vi "Hard.vi"() -> ()   [LabVIEW 2014]
uses:
  <vilib>/Utility/inputDevices.llb/keyboardAcquire.vi
  <vilib>/Utility/inputDevices.llb/closeKeyboard.vi
panel:
  out "Vx 2":i32
  out "x觸及位置 2":i32
  out "X障礙 2":bool
  out "y觸及位置 2":i32
  out "Vy 2":i32
  out "Y障礙 2":bool
  out "Å]YÄ²":i32
  out "Å]XÄ²":i32
  out "Å]Vy":i64
  out "Å]Vx":i32
  out "魔王":bool
  out "終點":bool
  out "遊玩時間":i32
  out "X障礙":bool
  out "Y位置 2":i32
  out "x位置 2":i32
  out "X":dbl
  out "Y":dbl
  out "小精靈":bool
  out "x位置":i32
  out "Y位置":i32
  out "Y障礙":bool
  out "x觸及位置":i32
  out "y觸及位置":i32
  out "x-y":u32
  out "Vy":i32
  out "Vx":i32
  # "小精靈"
  # "500"
  # "障礙"
  # "400"
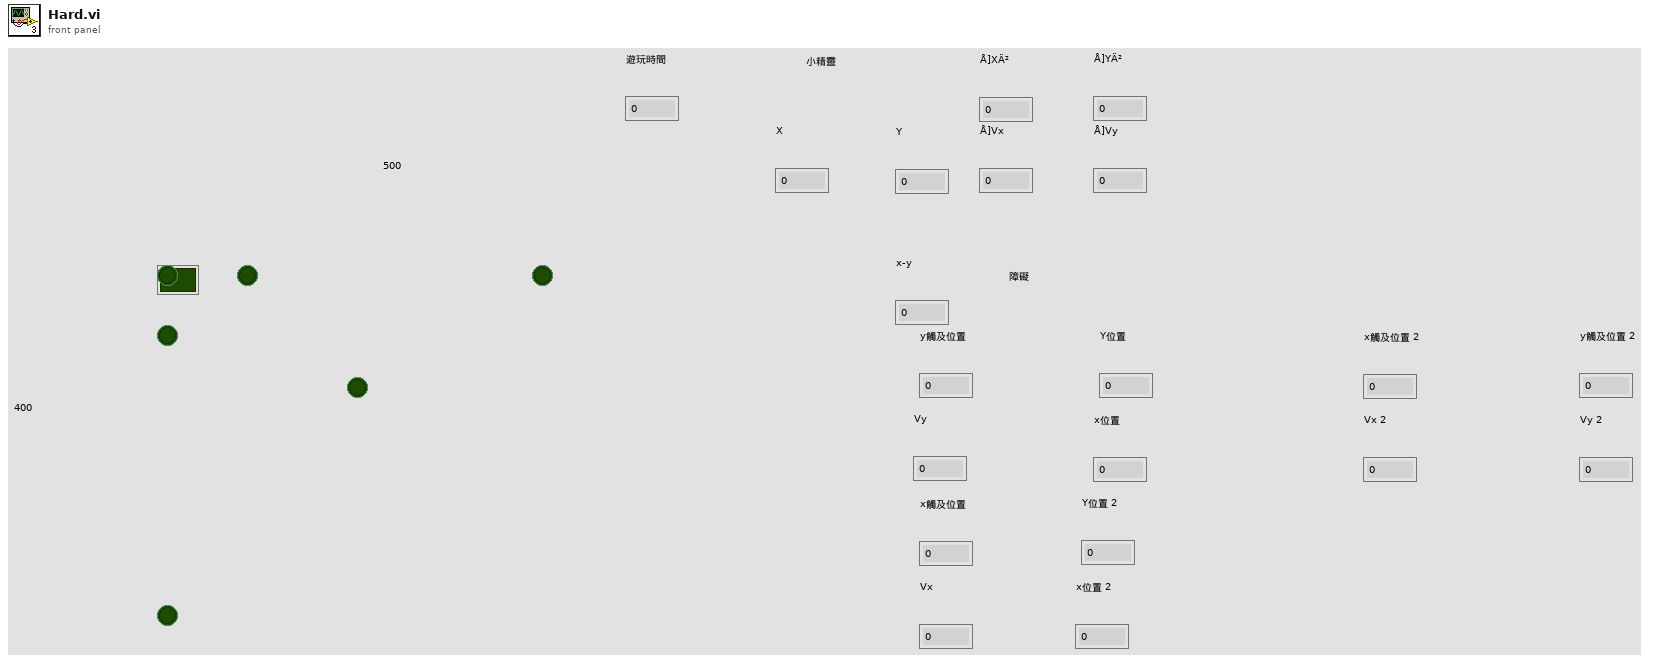
[diagram p1: front panel]
types:
  T1 = enum16{"0", "1", "2", "3", "4", "5", "6", "7", "8", "9", "A", "B", "C", "D", "E", "F", "G", "H", "I", "J", "K", "L", "M", "N", "O", "P", "Q", "R", "S", "T", "U", "V", "W", "X", "Y", "Z", "F1", "F2", "F3", "F4", "F5", "F6", "F7", "F8", "F9", "F10", "F11", "F12", "F13", "F14", "F15", "ADD", "BACK", "BACKSLASH", "CAPITAL", "COMMA", "DECIMAL", "DELETE", "DIVIDE", "DOWN", "END", "EQUALS", "ESCAPE", "GRAVE (`)", "HOME", "INSERT", "LBRACKET", "LCONTROL", "LEFT", "L ALT", "LSHIFT", "LWIN", "MINUS", "MULTIPLY", "NEXT", "NUMLOCK", "NUMPAD_0", "NUMPAD_1", "NUMPAD_2", "NUMPAD_3", "NUMPAD_4", "NUMPAD_5", "NUMPAD_6", "NUMPAD_7", "NUMPAD_8", "NUMPAD_9", "PAUSE", "PERIOD", "PRIOR (PG UP)", "RBRACKET", "RCONTROL", "RETURN", "RIGHT", "R ALT", "RSHIFT", "RWIN", "SCROLL", "SEMICOLON", "SLASH", "SPACE", "SUBTRACT", "TAB", "UP", "ENTER (num pad)", "' (quote)"}[]
  T2 = cluster{"keys pressed[0]":enum16{"0", "1", "2", "3", "4", "5", "6", "7", "8", "9", "A", "B", "C", "D", "E", "F", "G", "H", "I", "J", "K", "L", "M", "N", "O", "P", "Q", "R", "S", "T", "U", "V", "W", "X", "Y", "Z", "F1", "F2", "F3", "F4", "F5", "F6", "F7", "F8", "F9", "F10", "F11", "F12", "F13", "F14", "F15", "ADD", "BACK", "BACKSLASH", "CAPITAL", "COMMA", "DECIMAL", "DELETE", "DIVIDE", "DOWN", "END", "EQUALS", "ESCAPE", "GRAVE (`)", "HOME", "INSERT", "LBRACKET", "LCONTROL", "LEFT", "L ALT", "LSHIFT", "LWIN", "MINUS", "MULTIPLY", "NEXT", "NUMLOCK", "NUMPAD_0", "NUMPAD_1", "NUMPAD_2", "NUMPAD_3", "NUMPAD_4", "NUMPAD_5", "NUMPAD_6", "NUMPAD_7", "NUMPAD_8", "NUMPAD_9", "PAUSE", "PERIOD", "PRIOR (PG UP)", "RBRACKET", "RCONTROL", "RETURN", "RIGHT", "R ALT", "RSHIFT", "RWIN", "SCROLL", "SEMICOLON", "SLASH", "SPACE", "SUBTRACT", "TAB", "UP", "ENTER (num pad)", "' (quote)"}, "keys pressed[1]":enum16{"0", "1", "2", "3", "4", "5", "6", "7", "8", "9", "A", "B", "C", "D", "E", "F", "G", "H", "I", "J", "K", "L", "M", "N", "O", "P", "Q", "R", "S", "T", "U", "V", "W", "X", "Y", "Z", "F1", "F2", "F3", "F4", "F5", "F6", "F7", "F8", "F9", "F10", "F11", "F12", "F13", "F14", "F15", "ADD", "BACK", "BACKSLASH", "CAPITAL", "COMMA", "DECIMAL", "DELETE", "DIVIDE", "DOWN", "END", "EQUALS", "ESCAPE", "GRAVE (`)", "HOME", "INSERT", "LBRACKET", "LCONTROL", "LEFT", "L ALT", "LSHIFT", "LWIN", "MINUS", "MULTIPLY", "NEXT", "NUMLOCK", "NUMPAD_0", "NUMPAD_1", "NUMPAD_2", "NUMPAD_3", "NUMPAD_4", "NUMPAD_5", "NUMPAD_6", "NUMPAD_7", "NUMPAD_8", "NUMPAD_9", "PAUSE", "PERIOD", "PRIOR (PG UP)", "RBRACKET", "RCONTROL", "RETURN", "RIGHT", "R ALT", "RSHIFT", "RWIN", "SCROLL", "SEMICOLON", "SLASH", "SPACE", "SUBTRACT", "TAB", "UP", "ENTER (num pad)", "' (quote)"}, "keys pressed[2]":enum16{"0", "1", "2", "3", "4", "5", "6", "7", "8", "9", "A", "B", "C", "D", "E", "F", "G", "H", "I", "J", "K", "L", "M", "N", "O", "P", "Q", "R", "S", "T", "U", "V", "W", "X", "Y", "Z", "F1", "F2", "F3", "F4", "F5", "F6", "F7", "F8", "F9", "F10", "F11", "F12", "F13", "F14", "F15", "ADD", "BACK", "BACKSLASH", "CAPITAL", "COMMA", "DECIMAL", "DELETE", "DIVIDE", "DOWN", "END", "EQUALS", "ESCAPE", "GRAVE (`)", "HOME", "INSERT", "LBRACKET", "LCONTROL", "LEFT", "L ALT", "LSHIFT", "LWIN", "MINUS", "MULTIPLY", "NEXT", "NUMLOCK", "NUMPAD_0", "NUMPAD_1", "NUMPAD_2", "NUMPAD_3", "NUMPAD_4", "NUMPAD_5", "NUMPAD_6", "NUMPAD_7", "NUMPAD_8", "NUMPAD_9", "PAUSE", "PERIOD", "PRIOR (PG UP)", "RBRACKET", "RCONTROL", "RETURN", "RIGHT", "R ALT", "RSHIFT", "RWIN", "SCROLL", "SEMICOLON", "SLASH", "SPACE", "SUBTRACT", "TAB", "UP", "ENTER (num pad)", "' (quote)"}, "keys pressed[3]":enum16{"0", "1", "2", "3", "4", "5", "6", "7", "8", "9", "A", "B", "C", "D", "E", "F", "G", "H", "I", "J", "K", "L", "M", "N", "O", "P", "Q", "R", "S", "T", "U", "V", "W", "X", "Y", "Z", "F1", "F2", "F3", "F4", "F5", "F6", "F7", "F8", "F9", "F10", "F11", "F12", "F13", "F14", "F15", "ADD", "BACK", "BACKSLASH", "CAPITAL", "COMMA", "DECIMAL", "DELETE", "DIVIDE", "DOWN", "END", "EQUALS", "ESCAPE", "GRAVE (`)", "HOME", "INSERT", "LBRACKET", "LCONTROL", "LEFT", "L ALT", "LSHIFT", "LWIN", "MINUS", "MULTIPLY", "NEXT", "NUMLOCK", "NUMPAD_0", "NUMPAD_1", "NUMPAD_2", "NUMPAD_3", "NUMPAD_4", "NUMPAD_5", "NUMPAD_6", "NUMPAD_7", "NUMPAD_8", "NUMPAD_9", "PAUSE", "PERIOD", "PRIOR (PG UP)", "RBRACKET", "RCONTROL", "RETURN", "RIGHT", "R ALT", "RSHIFT", "RWIN", "SCROLL", "SEMICOLON", "SLASH", "SPACE", "SUBTRACT", "TAB", "UP", "ENTER (num pad)", "' (quote)"}, "keys pressed[4]":enum16{"0", "1", "2", "3", "4", "5", "6", "7", "8", "9", "A", "B", "C", "D", "E", "F", "G", "H", "I", "J", "K", "L", "M", "N", "O", "P", "Q", "R", "S", "T", "U", "V", "W", "X", "Y", "Z", "F1", "F2", "F3", "F4", "F5", "F6", "F7", "F8", "F9", "F10", "F11", "F12", "F13", "F14", "F15", "ADD", "BACK", "BACKSLASH", "CAPITAL", "COMMA", "DECIMAL", "DELETE", "DIVIDE", "DOWN", "END", "EQUALS", "ESCAPE", "GRAVE (`)", "HOME", "INSERT", "LBRACKET", "LCONTROL", "LEFT", "L ALT", "LSHIFT", "LWIN", "MINUS", "MULTIPLY", "NEXT", "NUMLOCK", "NUMPAD_0", "NUMPAD_1", "NUMPAD_2", "NUMPAD_3", "NUMPAD_4", "NUMPAD_5", "NUMPAD_6", "NUMPAD_7", "NUMPAD_8", "NUMPAD_9", "PAUSE", "PERIOD", "PRIOR (PG UP)", "RBRACKET", "RCONTROL", "RETURN", "RIGHT", "R ALT", "RSHIFT", "RWIN", "SCROLL", "SEMICOLON", "SLASH", "SPACE", "SUBTRACT", "TAB", "UP", "ENTER (num pad)", "' (quote)"}, "keys pressed[5]":enum16{"0", "1", "2", "3", "4", "5", "6", "7", "8", "9", "A", "B", "C", "D", "E", "F", "G", "H", "I", "J", "K", "L", "M", "N", "O", "P", "Q", "R", "S", "T", "U", "V", "W", "X", "Y", "Z", "F1", "F2", "F3", "F4", "F5", "F6", "F7", "F8", "F9", "F10", "F11", "F12", "F13", "F14", "F15", "ADD", "BACK", "BACKSLASH", "CAPITAL", "COMMA", "DECIMAL", "DELETE", "DIVIDE", "DOWN", "END", "EQUALS", "ESCAPE", "GRAVE (`)", "HOME", "INSERT", "LBRACKET", "LCONTROL", "LEFT", "L ALT", "LSHIFT", "LWIN", "MINUS", "MULTIPLY", "NEXT", "NUMLOCK", "NUMPAD_0", "NUMPAD_1", "NUMPAD_2", "NUMPAD_3", "NUMPAD_4", "NUMPAD_5", "NUMPAD_6", "NUMPAD_7", "NUMPAD_8", "NUMPAD_9", "PAUSE", "PERIOD", "PRIOR (PG UP)", "RBRACKET", "RCONTROL", "RETURN", "RIGHT", "R ALT", "RSHIFT", "RWIN", "SCROLL", "SEMICOLON", "SLASH", "SPACE", "SUBTRACT", "TAB", "UP", "ENTER (num pad)", "' (quote)"}, "keys pressed[6]":enum16{"0", "1", "2", "3", "4", "5", "6", "7", "8", "9", "A", "B", "C", "D", "E", "F", "G", "H", "I", "J", "K", "L", "M", "N", "O", "P", "Q", "R", "S", "T", "U", "V", "W", "X", "Y", "Z", "F1", "F2", "F3", "F4", "F5", "F6", "F7", "F8", "F9", "F10", "F11", "F12", "F13", "F14", "F15", "ADD", "BACK", "BACKSLASH", "CAPITAL", "COMMA", "DECIMAL", "DELETE", "DIVIDE", "DOWN", "END", "EQUALS", "ESCAPE", "GRAVE (`)", "HOME", "INSERT", "LBRACKET", "LCONTROL", "LEFT", "L ALT", "LSHIFT", "LWIN", "MINUS", "MULTIPLY", "NEXT", "NUMLOCK", "NUMPAD_0", "NUMPAD_1", "NUMPAD_2", "NUMPAD_3", "NUMPAD_4", "NUMPAD_5", "NUMPAD_6", "NUMPAD_7", "NUMPAD_8", "NUMPAD_9", "PAUSE", "PERIOD", "PRIOR (PG UP)", "RBRACKET", "RCONTROL", "RETURN", "RIGHT", "R ALT", "RSHIFT", "RWIN", "SCROLL", "SEMICOLON", "SLASH", "SPACE", "SUBTRACT", "TAB", "UP", "ENTER (num pad)", "' (quote)"}, "keys pressed[7]":enum16{"0", "1", "2", "3", "4", "5", "6", "7", "8", "9", "A", "B", "C", "D", "E", "F", "G", "H", "I", "J", "K", "L", "M", "N", "O", "P", "Q", "R", "S", "T", "U", "V", "W", "X", "Y", "Z", "F1", "F2", "F3", "F4", "F5", "F6", "F7", "F8", "F9", "F10", "F11", "F12", "F13", "F14", "F15", "ADD", "BACK", "BACKSLASH", "CAPITAL", "COMMA", "DECIMAL", "DELETE", "DIVIDE", "DOWN", "END", "EQUALS", "ESCAPE", "GRAVE (`)", "HOME", "INSERT", "LBRACKET", "LCONTROL", "LEFT", "L ALT", "LSHIFT", "LWIN", "MINUS", "MULTIPLY", "NEXT", "NUMLOCK", "NUMPAD_0", "NUMPAD_1", "NUMPAD_2", "NUMPAD_3", "NUMPAD_4", "NUMPAD_5", "NUMPAD_6", "NUMPAD_7", "NUMPAD_8", "NUMPAD_9", "PAUSE", "PERIOD", "PRIOR (PG UP)", "RBRACKET", "RCONTROL", "RETURN", "RIGHT", "R ALT", "RSHIFT", "RWIN", "SCROLL", "SEMICOLON", "SLASH", "SPACE", "SUBTRACT", "TAB", "UP", "ENTER (num pad)", "' (quote)"}, "keys pressed[8]":enum16{"0", "1", "2", "3", "4", "5", "6", "7", "8", "9", "A", "B", "C", "D", "E", "F", "G", "H", "I", "J", "K", "L", "M", "N", "O", "P", "Q", "R", "S", "T", "U", "V", "W", "X", "Y", "Z", "F1", "F2", "F3", "F4", "F5", "F6", "F7", "F8", "F9", "F10", "F11", "F12", "F13", "F14", "F15", "ADD", "BACK", "BACKSLASH", "CAPITAL", "COMMA", "DECIMAL", "DELETE", "DIVIDE", "DOWN", "END", "EQUALS", "ESCAPE", "GRAVE (`)", "HOME", "INSERT", "LBRACKET", "LCONTROL", "LEFT", "L ALT", "LSHIFT", "LWIN", "MINUS", "MULTIPLY", "NEXT", "NUMLOCK", "NUMPAD_0", "NUMPAD_1", "NUMPAD_2", "NUMPAD_3", "NUMPAD_4", "NUMPAD_5", "NUMPAD_6", "NUMPAD_7", "NUMPAD_8", "NUMPAD_9", "PAUSE", "PERIOD", "PRIOR (PG UP)", "RBRACKET", "RCONTROL", "RETURN", "RIGHT", "R ALT", "RSHIFT", "RWIN", "SCROLL", "SEMICOLON", "SLASH", "SPACE", "SUBTRACT", "TAB", "UP", "ENTER (num pad)", "' (quote)"}}
  T3 = enum16{"0", "1", "2", "3", "4", "5", "6", "7", "8", "9", "A", "B", "C", "D", "E", "F", "G", "H", "I", "J", "K", "L", "M", "N", "O", "P", "Q", "R", "S", "T", "U", "V", "W", "X", "Y", "Z", "F1", "F2", "F3", "F4", "F5", "F6", "F7", "F8", "F9", "F10", "F11", "F12", "F13", "F14", "F15", "ADD", "BACK", "BACKSLASH", "CAPITAL", "COMMA", "DECIMAL", "DELETE", "DIVIDE", "DOWN", "END", "EQUALS", "ESCAPE", "GRAVE (`)", "HOME", "INSERT", "LBRACKET", "LCONTROL", "LEFT", "L ALT", "LSHIFT", "LWIN", "MINUS", "MULTIPLY", "NEXT", "NUMLOCK", "NUMPAD_0", "NUMPAD_1", "NUMPAD_2", "NUMPAD_3", "NUMPAD_4", "NUMPAD_5", "NUMPAD_6", "NUMPAD_7", "NUMPAD_8", "NUMPAD_9", "PAUSE", "PERIOD", "PRIOR (PG UP)", "RBRACKET", "RCONTROL", "RETURN", "RIGHT", "R ALT", "RSHIFT", "RWIN", "SCROLL", "SEMICOLON", "SLASH", "SPACE", "SUBTRACT", "TAB", "UP", "ENTER (num pad)", "' (quote)"}
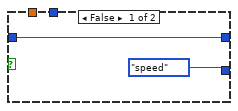
[diagram p3: hidden frame]
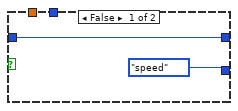
[diagram p5: hidden frame]
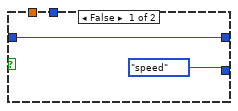
[diagram p7: hidden frame]
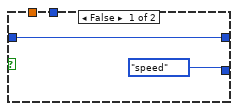
[diagram p13: hidden frame]
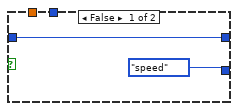
[diagram p15: hidden frame]
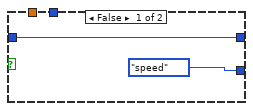
[diagram p17: hidden frame]
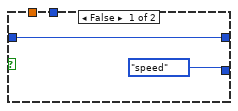
[diagram p19: hidden frame]
diagram:
  n1 = flat-sequence {
    tunnel: [w79] -> w26
    tunnel: [w78] -> w24
    tunnel: [w71] -> w12
    tunnel: [w70] -> w11
    tunnel: [w430] -> w27
    tunnel: w26 -> [w430]
    tunnel: [w429] -> w25
    tunnel: w24 -> [w429]
    tunnel: w12 -> [w408]
    tunnel: w11 -> [w409]
    tunnel: [w409] -> w10
    tunnel: [w408] -> w9
    tunnel: w27 -> [w465]
    tunnel: w25 -> [w464]
    tunnel: [w455] -> w21
    tunnel: [w454] -> w19
    tunnel: [w453] -> w17
    tunnel: [w452] -> w15
    tunnel: [w451] -> w13
    tunnel: w10 -> [w444]
    tunnel: w9 -> [w443]
    tunnel: [w442] -> w8
    tunnel: [w441] -> w7
    tunnel: [w440] -> w4
    tunnel: [w439] -> w3
    tunnel: [w952] -> w22
    tunnel: w21 -> [w952]
    tunnel: [w951] -> w20
    tunnel: w19 -> [w951]
    tunnel: [w950] -> w18
    tunnel: w17 -> [w950]
    tunnel: [w949] -> w16
    tunnel: w15 -> [w949]
    tunnel: [w948] -> w14
    tunnel: w13 -> [w948]
    tunnel: w8 -> [w933]
    tunnel: w7 -> [w932]
    tunnel: [w933] -> w6
    tunnel: [w932] -> w5
    tunnel: w4 -> [w931]
    tunnel: w3 -> [w930]
    tunnel: [w931] -> w2
    tunnel: [w930] -> w1
    tunnel: w22 -> [w984]
    tunnel: w20 -> [w983]
    tunnel: w18 -> [w982]
    tunnel: w16 -> [w981]
    tunnel: w14 -> [w980]
    tunnel: w6 -> [w962]
    tunnel: w5 -> [w961]
    tunnel: w2 -> [w960]
    tunnel: w1 -> [w959]
    frame #0 {
      # "下:小精靈控制"
      # "上:障礙控制"
      n2 = Random Number (0-1)() -> (number: 0 to 1=w59:dbl)
      n3 = Random Number (0-1)() -> (number: 0 to 1=w64:dbl)
      n4 = Multiply(x=200.0, y=w59) -> (x*y=w57:dbl)
      n5 = Random Number (0-1)() -> (number: 0 to 1=w33:dbl)
      n6 = property on="Y障礙 2" class="Bool (strict)"("Left"=300 ("Position:Left"), "Top"=1 ("Position:Top")) -> ()  [unwired: 2 in, 2 out]
      n7 = Random Number (0-1)() -> (number: 0 to 1=w41:dbl)
      n8 = property on="Y障礙" class="Bool (strict)"("Left"=200 ("Position:Left"), "Top"=1 ("Position:Top")) -> ()  [unwired: 2 in, 2 out]
      n9 = property on="魔王" class="Bool (strict)"("Left"=-500 ("Position:Left"), "Top"=0 ("Position:Top")) -> ()  [unwired: 2 in, 2 out]
      n10 = Add(x=100.0 ("Vy"), y=w57) -> (x+y=→"Vy":dbl)
      n11 = Multiply(x=200.0, y=w33) -> (x*y=w31:dbl)
      n12 = Multiply(x=200.0, y=w64) -> (x*y=w62:dbl)
      n13 = Add(x=100.0 ("y"), y=w62) -> (x+y=→"Vx":dbl)
      n14 = Add(x=100.0 ("Vy"), y=w31) -> (x+y=→"Vy 2":dbl)
      n15 = Multiply(x=200.0, y=w41) -> (x*y=w39:dbl)
      n16 = Add(x=100.0 ("y"), y=w39) -> (x+y=→"Vx 2":dbl)
      n17 = property on="小精靈" class="Bool (strict)"("Left"=0 ("Position:Left"), "Top"=0 ("Position:Top")) -> ()  [unwired: 2 in, 2 out]
      n18 = property on="終點" class="Bool (strict)"("Left"=477 ("Position:Left"), "Top"=374 ("Position:Top")) -> ()  [unwired: 2 in, 2 out]
      n19 = property on="X障礙" class="Bool (strict)"("Left"=1 ("Position:Left"), "Top"=200 ("Position:Top")) -> ()  [unwired: 2 in, 2 out]
      n20 = property on="X障礙 2" class="Bool (strict)"("Left"=1 ("Position:Left"), "Top"=270 ("Position:Top")) -> ()  [unwired: 2 in, 2 out]
      "y觸及位置" <- 0.0 ("x*y")
      "x觸及位置" <- 0.0 ("x*y")
      "小精靈" <- TRUE
      "X" <- 0.0 ("Numeric")
      "Y" <- 0.0 ("Y")
      "遊玩時間" <- 0 ("Numeric")
      "x觸及位置 2" <- 0.0 ("x*y")
      "y觸及位置 2" <- 0.0 ("x*y")
    }
    frame #1 {
      w74 = 0 ("Left")
      w75 = 0 ("Left")
      w80 = 0
      w81 = 0
      n21 = call <vilib>:"Intialize Keyboard.vi"() -> ("error out"=w85:errorcluster, "device ID"=w87:refnum<k1>)  [unwired: 10 in]
      n22 = Tick Count (ms)() -> (millisecond timer value=w88:u32)
      n23 = Tick Count (ms)() -> (millisecond timer value=w83:u32)
      n24 = Tick Count (ms)() -> (millisecond timer value=w73:u32)
      n25 = Tick Count (ms)() -> (millisecond timer value=w77:u32)
      n26 = while {
        shift-right: [w198] -> _
        shift-left: enum16{"speed"}."speed" ("Enum") -> [w200]
        shift-right: [w199] -> _
        shift-left: w88 -> [w201]
        tunnel: w87 -> [w197]
        tunnel: [w164] -> w86
        tunnel: w85 -> [w196]
        tunnel: [w163] -> w84
        shift-right: [w192] -> _
        shift-left: w83 -> [w193]
        shift-right: [w191] -> _
        shift-left: enum16{"speed"}."speed" ("Enum") -> [w190]
        shift-right: [w187] -> _
        shift-left: w81 -> [w185]
        shift-left: w81 -> [w184]
        shift-right: [w186] -> _
        shift-left: w80 -> [w183]
        shift-left: w80 -> [w182]
        tunnel: [w145] -> w79
        tunnel: [w144] -> w78
        shift-right: [w134] -> _
        shift-left: w77 -> [w136]
        shift-right: [w135] -> _
        shift-left: enum16{"speed"}."speed" ("Enum") -> [w137]
        shift-right: [w133] -> _
        shift-left: w75 -> [w132]
        shift-left: w75 -> [w131]
        shift-right: [w130] -> _
        shift-left: w74 -> [w129]
        shift-left: w74 -> [w128]
        shift-right: [w125] -> _
        shift-left: w73 -> [w127]
        shift-right: [w124] -> _
        shift-left: enum16{"speed"}."speed" ("Enum") -> [w126]
        tunnel: [w90] -> w71
        tunnel: [w91] -> w70
        stop <- w143 stop-if-true
        n27 = local read "遊玩時間"() -> (w142:i32)
        n28 = case shown="\"speed\"" w190 {
          tunnel: w193 -> [w323]
          tunnel: [w322] -> w192
          tunnel: [w321] -> w191
          tunnel: w185 -> [w311]
          tunnel: w184 -> [w310]
          tunnel: w185 -> [w305]
          tunnel: w184 -> [w304]
          tunnel: [w299] -> w187
          tunnel: w185 -> [_]
          tunnel: w184 -> [_]
          frame "speed" {
            n29 = Tick Count (ms)() -> (millisecond timer value=w332:u32)
            n30 = Greater?(x=w311, y=500.0) -> (0:w307:bool)
            n31 = Greater?(x=w310, y=500.0) -> (0:w306:bool)
            n32 = Less?(x=w305, y=0.0) -> (x < y?=w301:bool)
            n33 = Less?(x=w304, y=0.0) -> (x < y?=w300:bool)
            n34 = property on="X障礙" class="Bool (strict)"() -> ("Left"=w324:i32)  [unwired: 2 in, 2 out]
            n35 = property on="X障礙" class="Bool (strict)"() -> ("Left"=w318:i32)  [unwired: 2 in, 2 out]
            n36 = Less?(x=w318, y=0) -> (x < y?=w316:bool)
            n37 = Greater?(x=w324, y=500) -> (0:w315:bool)
            n38 = And(x=w307, y=w306) -> (x .and. y?=w298:bool)
            n39 = And(x=w301, y=w300) -> (x .and. y?=w297:bool)
            n40 = Subtract(x=w332, y=w323) -> (x-y=w331:u32)
            n41 = Or(x=w315, y=w316) -> (x .or. y?=w314:bool)
            n42 = To Double Precision Float(number=w331) -> (double precision float=w330:dbl)
            n43 = Compound Arithmetic op=OR(w298, w297) -> (w296:bool)
            n44 = local read "Vx"() -> (w320:i32)
            n45 = local read "x觸及位置"() -> (w326:i32)
            n46 = Divide(x=w330, y=1000.0) -> (x/y=w328:dbl)
            n47 = case shown="True" w296 {
              frame False {
              }
              frame True {
                w333 = 200 ("x觸及位置")
                n48 = local write "x觸及位置"(w333) -> ()
                n49 = Wait (ms)(milliseconds to wait=u32 100) -> ()  [unwired: 1 out]
                n50 = property on="X障礙" class="Bool (strict)"("Left"=w333) -> ()  [unwired: 2 in, 2 out]
              }
            }
            n51 = Multiply(x=w328, y=w320) -> (x*y=w327:dbl)
            n52 = Add(x=w327, y=w326) -> (x+y=w312:dbl)
            n53 = case shown="True" w314 {
              tunnel: [enum16{"speed"}."speed" ("Enum") enum16{"speed"}."speed" ("Enum")] -> w321
              tunnel: [w335 w342] -> w322
              tunnel: w323 -> [w335 _]
              tunnel: w312 -> [_ w339]
              tunnel: w320 -> [_ w341]
              frame False {
              }
              frame True {
                n54 = local write "x觸及位置"(w339) -> ()
                n55 = Multiply(x=w341, y=-1.0) -> (x*y=w338:dbl)
                n56 = Wait (ms)(milliseconds to wait=u32 25) -> ()  [unwired: 1 out]
                n57 = Tick Count (ms)() -> (millisecond timer value=w342:u32)
                n58 = local write "Vx"(w338) -> ()
              }
            }
            n59 = property on="X障礙" class="Bool (strict)"("Left"=w312) -> ()  [unwired: 2 in, 2 out]
            n60 = property on="X障礙" class="Bool (strict)"() -> ("Top"=→"Y位置 2":i32, "Left"=w299:i32)  [unwired: 2 in, 2 out]
            "x位置 2" <- w299
            n61 = Wait (ms)(milliseconds to wait=u32 10) -> ()  [unwired: 1 out]
          }
        }
        n62 = case shown="\"speed\"" w137 {
          tunnel: w136 -> [w275]
          tunnel: [w274] -> w134
          tunnel: [w273] -> w135
          tunnel: w132 -> [w264]
          tunnel: w131 -> [w263]
          tunnel: w132 -> [w258]
          tunnel: w131 -> [w257]
          tunnel: [w249] -> w133
          frame "speed" {
            n63 = Tick Count (ms)() -> (millisecond timer value=w284:u32)
            n64 = Greater?(x=w264, y=500.0) -> (0:w260:bool)
            n65 = Greater?(x=w263, y=500.0) -> (0:w259:bool)
            n66 = Less?(x=w258, y=0.0) -> (x < y?=w254:bool)
            n67 = Less?(x=w257, y=0.0) -> (x < y?=w253:bool)
            n68 = property on="X障礙 2" class="Bool (strict)"() -> ("Left"=w276:i32)  [unwired: 2 in, 2 out]
            n69 = property on="X障礙 2" class="Bool (strict)"() -> ("Left"=w270:i32)  [unwired: 2 in, 2 out]
            n70 = Less?(x=w270, y=0) -> (x < y?=w268:bool)
            n71 = Greater?(x=w276, y=500) -> (0:w267:bool)
            n72 = And(x=w260, y=w259) -> (x .and. y?=w252:bool)
            n73 = And(x=w254, y=w253) -> (x .and. y?=w251:bool)
            n74 = Subtract(x=w284, y=w275) -> (x-y=w283:u32)
            n75 = Or(x=w267, y=w268) -> (x .or. y?=w266:bool)
            n76 = To Double Precision Float(number=w283) -> (double precision float=w282:dbl)
            n77 = Compound Arithmetic op=OR(w252, w251) -> (w250:bool)
            n78 = local read "Vx 2"() -> (w272:i32)
            n79 = local read "x觸及位置 2"() -> (w278:i32)
            n80 = Divide(x=w282, y=1000.0) -> (x/y=w280:dbl)
            n81 = case shown="True" w250 {
              frame False {
              }
              frame True {
                w285 = 200 ("x觸及位置")
                n82 = local write "x觸及位置 2"(w285) -> ()
                n83 = property on="X障礙 2" class="Bool (strict)"("Left"=w285) -> ()  [unwired: 2 in, 2 out]
                n84 = Wait (ms)(milliseconds to wait=u32 100) -> ()  [unwired: 1 out]
              }
            }
            n85 = Multiply(x=w280, y=w272) -> (x*y=w279:dbl)
            n86 = Add(x=w279, y=w278) -> (x+y=w265:dbl)
            n87 = case shown="True" w266 {
              tunnel: [enum16{"speed"}."speed" ("Enum") enum16{"speed"}."speed" ("Enum")] -> w273
              tunnel: [w287 w294] -> w274
              tunnel: w275 -> [w287 _]
              tunnel: w265 -> [_ w291]
              tunnel: w272 -> [_ w293]
              frame False {
              }
              frame True {
                n88 = local write "x觸及位置 2"(w291) -> ()
                n89 = Multiply(x=w293, y=-1.0) -> (x*y=w290:dbl)
                n90 = Wait (ms)(milliseconds to wait=u32 25) -> ()  [unwired: 1 out]
                n91 = local write "Vx 2"(w290) -> ()
                n92 = Tick Count (ms)() -> (millisecond timer value=w294:u32)
              }
            }
            n93 = property on="X障礙 2" class="Bool (strict)"("Left"=w265) -> ()  [unwired: 2 in, 2 out]
            n94 = property on="X障礙 2" class="Bool (strict)"() -> ("Left"=w249:i32)  [unwired: 2 in, 2 out]
            n95 = Wait (ms)(milliseconds to wait=u32 10) -> ()  [unwired: 1 out]
          }
        }
        n96 = case shown="\"speed\"" w126 {
          tunnel: w127 -> [w228]
          tunnel: [w227] -> w125
          tunnel: [w226] -> w124
          tunnel: w129 -> [w217]
          tunnel: w128 -> [w216]
          tunnel: w129 -> [w211]
          tunnel: w128 -> [w210]
          tunnel: [w202] -> w130
          frame "speed" {
            n97 = Tick Count (ms)() -> (millisecond timer value=w237:u32)
            n98 = Greater?(x=w217, y=400.0) -> (0:w213:bool)
            n99 = Greater?(x=w216, y=400.0) -> (0:w212:bool)
            n100 = Less?(x=w211, y=0.0) -> (x < y?=w207:bool)
            n101 = Less?(x=w210, y=0.0) -> (x < y?=w206:bool)
            n102 = property on="Y障礙 2" class="Bool (strict)"() -> ("Top"=w229:i32)  [unwired: 2 in, 2 out]
            n103 = property on="Y障礙 2" class="Bool (strict)"() -> ("Top"=w223:i32)  [unwired: 2 in, 2 out]
            n104 = Less?(x=w223, y=0) -> (x < y?=w221:bool)
            n105 = Greater?(x=w229, y=400) -> (0:w220:bool)
            n106 = And(x=w213, y=w212) -> (x .and. y?=w205:bool)
            n107 = And(x=w207, y=w206) -> (x .and. y?=w204:bool)
            n108 = Subtract(x=w237, y=w228) -> (x-y=w236:u32)
            n109 = Or(x=w220, y=w221) -> (x .or. y?=w219:bool)
            n110 = To Double Precision Float(number=w236) -> (double precision float=w235:dbl)
            n111 = Compound Arithmetic op=OR(w205, w204) -> (w203:bool)
            n112 = local read "Vy 2"() -> (w225:i32)
            n113 = local read "y觸及位置 2"() -> (w231:i32)
            n114 = Divide(x=w235, y=1000.0) -> (x/y=w233:dbl)
            n115 = case shown="True" w203 {
              frame False {
              }
              frame True {
                w238 = 200 ("x觸及位置")
                n116 = local write "y觸及位置 2"(w238) -> ()
                n117 = property on="Y障礙 2" class="Bool (strict)"("Top"=w238) -> ()  [unwired: 2 in, 2 out]
                n118 = Wait (ms)(milliseconds to wait=u32 100) -> ()  [unwired: 1 out]
              }
            }
            n119 = Multiply(x=w233, y=w225) -> (x*y=w232:dbl)
            n120 = Add(x=w232, y=w231) -> (x+y=w218:dbl)
            n121 = case shown="True" w219 {
              tunnel: [enum16{"speed"}."speed" ("Enum") enum16{"speed"}."speed" ("Enum")] -> w226
              tunnel: [w240 w247] -> w227
              tunnel: w228 -> [w240 _]
              tunnel: w218 -> [_ w244]
              tunnel: w225 -> [_ w246]
              frame False {
              }
              frame True {
                n122 = local write "y觸及位置 2"(w244) -> ()
                n123 = Multiply(x=w246, y=-1.0) -> (x*y=w243:dbl)
                n124 = Wait (ms)(milliseconds to wait=u32 25) -> ()  [unwired: 1 out]
                n125 = local write "Vy 2"(w243) -> ()
                n126 = Tick Count (ms)() -> (millisecond timer value=w247:u32)
              }
            }
            n127 = property on="Y障礙 2" class="Bool (strict)"("Top"=w218) -> ()  [unwired: 2 in, 2 out]
            n128 = property on="Y障礙 2" class="Bool (strict)"() -> ("Top"=w202:i32)  [unwired: 2 in, 2 out]
            n129 = Wait (ms)(milliseconds to wait=u32 10) -> ()  [unwired: 1 out]
          }
        }
        n130 = Increment(x=w142) -> (x+1=w141:i32)
        n131 = property on="X障礙 2" class="Bool (strict)"() -> ("Top"=w92:i32)  [unwired: 2 in, 2 out]
        n132 = property on="X障礙 2" class="Bool (strict)"() -> ("Top"=w98:i32)  [unwired: 2 in, 2 out]
        n133 = property on="X障礙 2" class="Bool (strict)"() -> ("Left"=w105:i32)  [unwired: 2 in, 2 out]
        n134 = property on="X障礙 2" class="Bool (strict)"() -> ("Left"=w103:i32)  [unwired: 2 in, 2 out]
        n135 = call-poly <vilib>:"Acquire Input Data.vi"("device ID"=w197, "error in (no error)"=w196) -> ("device ID"=w164:refnum<k1>, "keys pressed"=w195:T1, "error out"=w163:errorcluster)  [unwired: 15 in]
        n136 = case shown="\"speed\"" w200 {
          tunnel: w201 -> [w387]
          tunnel: [w386] -> w199
          tunnel: [w385] -> w198
          tunnel: w183 -> [w367]
          tunnel: w183 -> [w366]
          tunnel: w182 -> [w365]
          tunnel: w182 -> [w364]
          tunnel: [w363] -> w186
          tunnel: w183 -> [_]
          tunnel: w182 -> [_]
          frame "speed" {
            n137 = Tick Count (ms)() -> (millisecond timer value=w396:u32)
            n138 = property on="Y障礙" class="Bool (strict)"() -> ("Top"=w388:i32)  [unwired: 2 in, 2 out]
            n139 = property on="Y障礙" class="Bool (strict)"() -> ("Top"=w382:i32)  [unwired: 2 in, 2 out]
            n140 = Less?(x=w382, y=0) -> (x < y?=w380:bool)
            n141 = Greater?(x=w388, y=400) -> (0:w379:bool)
            n142 = Subtract(x=w396, y=w387) -> (x-y=w395:u32)
            "x-y" <- w395
            n143 = Greater?(x=w367, y=400.0) -> (0:w373:bool)
            n144 = Greater?(x=w365, y=400.0) -> (0:w372:bool)
            n145 = Less?(x=w366, y=0.0) -> (x < y?=w369:bool)
            n146 = Less?(x=w364, y=0.0) -> (x < y?=w368:bool)
            n147 = Or(x=w379, y=w380) -> (x .or. y?=w378:bool)
            n148 = To Double Precision Float(number=w395) -> (double precision float=w394:dbl)
            n149 = And(x=w373, y=w372) -> (x .and. y?=w362:bool)
            n150 = And(x=w369, y=w368) -> (x .and. y?=w361:bool)
            n151 = local read "Vy"() -> (w384:i32)
            n152 = local read "y觸及位置"() -> (w390:i32)
            n153 = Divide(x=w394, y=1000.0) -> (x/y=w392:dbl)
            n154 = Compound Arithmetic op=OR(w362, w361) -> (w360:bool)
            n155 = case shown="True" w360 {
              frame False {
              }
              frame True {
                w397 = 200 ("y觸及位置")
                n156 = local write "y觸及位置"(w397) -> ()
                n157 = Wait (ms)(milliseconds to wait=u32 100) -> ()  [unwired: 1 out]
                n158 = property on="Y障礙" class="Bool (strict)"("Top"=w397) -> ()  [unwired: 2 in, 2 out]
              }
            }
            n159 = Multiply(x=w392, y=w384) -> (x*y=w391:dbl)
            n160 = Add(x=w391, y=w390) -> (x+y=w376:dbl)
            n161 = case shown="True" w378 {
              tunnel: [enum16{"speed"}."speed" ("Enum") enum16{"speed"}."speed" ("Enum")] -> w385
              tunnel: [w399 w406] -> w386
              tunnel: w387 -> [w399 _]
              tunnel: w376 -> [_ w402]
              tunnel: w384 -> [_ w404]
              frame False {
              }
              frame True {
                n162 = local write "y觸及位置"(w402) -> ()
                n163 = Multiply(x=w404, y=-1.0) -> (x*y=w401:dbl)
                n164 = Wait (ms)(milliseconds to wait=u32 25) -> ()  [unwired: 1 out]
                n165 = Tick Count (ms)() -> (millisecond timer value=w406:u32)
                n166 = local write "Vy"(w401) -> ()
              }
            }
            n167 = property on="Y障礙" class="Bool (strict)"("Top"=w376) -> ()  [unwired: 2 in, 2 out]
            n168 = Wait (ms)(milliseconds to wait=u32 10) -> ()  [unwired: 1 out]
            n169 = property on="Y障礙" class="Bool (strict)"() -> ("Top"=w363:i32, "Left"=→"x位置":i32)  [unwired: 2 in, 2 out]
            "Y位置" <- w363
          }
        }
        n170 = local write "遊玩時間"(w141) -> ()
        n171 = local read "Y"() -> (w106:dbl)
        n172 = local read "X"() -> (w107:dbl)
        n173 = Array To Cluster(array=w195) -> (cluster=w165:T2)
        n174 = Unbundle(w165) -> ("keys pressed[0]"=w194:T3)  [unwired: 8 out]
        n175 = case shown="\"A\"" w194 {
          frame Default {
          }
          frame "A" {
            n176 = local read "X"() -> (w358:dbl)
            n177 = Wait (ms)(milliseconds to wait=u32 10) -> ()  [unwired: 1 out]
            n178 = Add(x=-2.0, y=w358) -> (x+y=w356:dbl)
            n179 = local write "X"(w356) -> ()
            n180 = property on="小精靈" class="Bool (strict)"("Left"=w356) -> ()  [unwired: 2 in, 2 out]
          }
        }
        n181 = case shown="\"D\"" w194 {
          frame Default {
          }
          frame "D" {
            n182 = local read "X"() -> (w354:dbl)
            n183 = Wait (ms)(milliseconds to wait=u32 10) -> ()  [unwired: 1 out]
            n184 = Add(x=2.0, y=w354) -> (x+y=w352:dbl)
            n185 = local write "X"(w352) -> ()
            n186 = property on="小精靈" class="Bool (strict)"("Left"=w352) -> ()  [unwired: 2 in, 2 out]
          }
        }
        n187 = Add(x=w105, y=17) -> (x+y=w100:i32)
        n188 = Subtract(x=w103, y=17) -> (x-y=w101:i32)
        n189 = Subtract(x=w98, y=15) -> (x-y=w97:i32)
        n190 = Add(x=w92, y=20) -> (x+y=w93:i32)
        n191 = property on="X障礙" class="Bool (strict)"() -> ("Top"=w162:i32)  [unwired: 2 in, 2 out]
        n192 = property on="X障礙" class="Bool (strict)"() -> ("Top"=w156:i32)  [unwired: 2 in, 2 out]
        n193 = property on="X障礙" class="Bool (strict)"() -> ("Left"=w149:i32)  [unwired: 2 in, 2 out]
        n194 = property on="X障礙" class="Bool (strict)"() -> ("Left"=w151:i32)  [unwired: 2 in, 2 out]
        n195 = In Range and Coerce(upper limit=w100, x=w107, lower limit=w101) -> (In Range?=w96:bool)  [unwired: 1 out]
        n196 = In Range and Coerce(upper limit=w93, x=w106, lower limit=w97) -> (In Range?=w95:bool)  [unwired: 1 out]
        n197 = local read "Y"() -> (w148:dbl)
        n198 = local read "X"() -> (w147:dbl)
        n199 = And(x=w96, y=w95) -> (x .and. y?=w91:bool)
        n200 = Add(x=w149, y=17) -> (x+y=w154:i32)
        n201 = Subtract(x=w151, y=17) -> (x-y=w153:i32)
        n202 = Subtract(x=w156, y=15) -> (x-y=w157:i32)
        n203 = Add(x=w162, y=20) -> (x+y=w161:i32)
        n204 = property on="小精靈" class="Bool (strict)"() -> ("Left"=w189:i32)  [unwired: 2 in, 2 out]
        n205 = property on="Y障礙 2" class="Bool (strict)"() -> ("Top"=w123:i32)  [unwired: 2 in, 2 out]
        n206 = property on="Y障礙 2" class="Bool (strict)"() -> ("Top"=w117:i32)  [unwired: 2 in, 2 out]
        n207 = property on="Y障礙 2" class="Bool (strict)"() -> ("Left"=w110:i32)  [unwired: 2 in, 2 out]
        n208 = property on="Y障礙 2" class="Bool (strict)"() -> ("Left"=w112:i32)  [unwired: 2 in, 2 out]
        n209 = In Range and Coerce(upper limit=w154, x=w147, lower limit=w153) -> (In Range?=w158:bool)  [unwired: 1 out]
        n210 = In Range and Coerce(upper limit=w161, x=w148, lower limit=w157) -> (In Range?=w159:bool)  [unwired: 1 out]
        n211 = local read "Y"() -> (w109:dbl)
        n212 = local read "X"() -> (w108:dbl)
        n213 = And(x=w158, y=w159) -> (x .and. y?=w144:bool)
        n214 = local read "遊玩時間"() -> (w140:i32)
        n215 = Add(x=w110, y=17) -> (x+y=w115:i32)
        n216 = Subtract(x=w112, y=17) -> (x-y=w114:i32)
        n217 = Subtract(x=w117, y=15) -> (x-y=w118:i32)
        n218 = Add(x=w123, y=20) -> (x+y=w122:i32)
        n219 = case shown="\"W\"" w194 {
          frame Default {
          }
          frame "W" {
            n220 = local read "Y"() -> (w350:dbl)
            n221 = Wait (ms)(milliseconds to wait=u32 10) -> ()  [unwired: 1 out]
            n222 = Add(x=-2.0, y=w350) -> (x+y=w348:dbl)
            n223 = local write "Y"(w348) -> ()
            n224 = property on="小精靈" class="Bool (strict)"("Top"=w348) -> ()  [unwired: 2 in, 2 out]
          }
        }
        n225 = case shown="\"S\"" w194 {
          frame Default {
          }
          frame "S" {
            n226 = local read "Y"() -> (w346:dbl)
            n227 = Wait (ms)(milliseconds to wait=u32 10) -> ()  [unwired: 1 out]
            n228 = Add(x=2.0, y=w346) -> (x+y=w344:dbl)
            n229 = local write "Y"(w344) -> ()
            n230 = property on="小精靈" class="Bool (strict)"("Top"=w344) -> ()  [unwired: 2 in, 2 out]
          }
        }
        n231 = property on="Y障礙" class="Bool (strict)"() -> ("Top"=w166:i32)  [unwired: 2 in, 2 out]
        n232 = property on="Y障礙" class="Bool (strict)"() -> ("Top"=w172:i32)  [unwired: 2 in, 2 out]
        n233 = property on="Y障礙" class="Bool (strict)"() -> ("Left"=w179:i32)  [unwired: 2 in, 2 out]
        n234 = property on="Y障礙" class="Bool (strict)"() -> ("Left"=w177:i32)  [unwired: 2 in, 2 out]
        n235 = Greater?(x=w189, y=250) -> (0:w146:bool)
        n236 = local read "Y"() -> (w180:dbl)
        n237 = In Range and Coerce(upper limit=w115, x=w108, lower limit=w114) -> (In Range?=w119:bool)  [unwired: 1 out]
        n238 = In Range and Coerce(upper limit=w122, x=w109, lower limit=w118) -> (In Range?=w120:bool)  [unwired: 1 out]
        n239 = local read "X"() -> (w181:dbl)
        n240 = Greater?(x=w140, y=500) -> (0:w138:bool)
        n241 = And(x=w119, y=w120) -> (x .and. y?=w90:bool)
        n242 = Add(x=w179, y=17) -> (x+y=w174:i32)
        n243 = Subtract(x=w177, y=17) -> (x-y=w175:i32)
        n244 = Subtract(x=w172, y=15) -> (x-y=w171:i32)
        n245 = Add(x=w166, y=20) -> (x+y=w167:i32)
        n246 = In Range and Coerce(upper limit=w174, x=w181, lower limit=w175) -> (In Range?=w170:bool)  [unwired: 1 out]
        n247 = In Range and Coerce(upper limit=w167, x=w180, lower limit=w171) -> (In Range?=w169:bool)  [unwired: 1 out]
        n248 = And(x=w170, y=w169) -> (x .and. y?=w145:bool)
        n249 = Compound Arithmetic op=OR(w138, w146, w144, w145, w91, w90) -> (w143:bool)
      }
      n250 = call-poly <vilib>:"Close Input Device.vi"("error in (no error)"=w84, "device ID"=w86) -> ()  [unwired: 8 in, 1 out]
    }
    frame #2 {
      w418 = 0.0 ("x*y")
      n251 = Random Number (0-1)() -> (number: 0 to 1=w423:dbl)
      n252 = Random Number (0-1)() -> (number: 0 to 1=w427:dbl)
      n253 = property on="Y障礙" class="Bool (strict)"("Left"=375 ("Position:Left"), "Top"=1 ("Position:Top")) -> ()  [unwired: 2 in, 2 out]
      n254 = property on="Y障礙 2" class="Bool (strict)"("Left"=300 ("Position:Left"), "Top"=1 ("Position:Top")) -> ()  [unwired: 2 in, 2 out]
      n255 = local write "x觸及位置 2"(0 ("x觸及位置")) -> ()
      n256 = local write "Vy"(300 ("Vy")) -> ()
      n257 = local write "Vx"(300 ("Vx")) -> ()
      n258 = Multiply(x=200.0, y=w423) -> (x*y=w421:dbl)
      n259 = Add(x=300.0 ("y"), y=w421) -> (x+y=→"Å]Vy":dbl)
      n260 = local write "y觸及位置 2"(0 ("y觸及位置")) -> ()
      n261 = local write "y觸及位置"(0 ("y觸及位置")) -> ()
      n262 = local write "x觸及位置"(0 ("x觸及位置")) -> ()
      n263 = Multiply(x=200.0, y=w427) -> (x*y=w425:dbl)
      n264 = Add(x=300.0 ("y"), y=w425) -> (x+y=→"Å]Vx":dbl)
      n265 = property on="X障礙 2" class="Bool (strict)"("Left"=1 ("Position:Left"), "Top"=270 ("Position:Top")) -> ()  [unwired: 2 in, 2 out]
      n266 = property on="X障礙" class="Bool (strict)"("Left"=1 ("Position:Left"), "Top"=340 ("Position:Top")) -> ()  [unwired: 2 in, 2 out]
      n267 = local write "Vx 2"(300 ("Vx 2")) -> ()
      n268 = local write "Vy 2"(270 ("Vy 2")) -> ()
      "Å]XÄ²" <- w418
      "Å]YÄ²" <- w418
    }
    frame #3 {
      w446 = 0 ("Left")
      w445 = 0 ("Top")
      w456 = 0
      w457 = 0
      w466 = 0 ("Top")
      w467 = 0
      n269 = Tick Count (ms)() -> (millisecond timer value=w469:u32)
      n270 = Tick Count (ms)() -> (millisecond timer value=w460:u32)
      n271 = Tick Count (ms)() -> (millisecond timer value=w449:u32)
      n272 = Tick Count (ms)() -> (millisecond timer value=w448:u32)
      n273 = call <vilib>:"Intialize Keyboard.vi"() -> ("error out"=w470:errorcluster, "device ID"=w471:refnum<k1>)  [unwired: 10 in]
      n274 = Tick Count (ms)() -> (millisecond timer value=w459:u32)
      n275 = Tick Count (ms)() -> (millisecond timer value=w472:u32)
      n276 = while {
        shift-right: [w620] -> _
        shift-left: enum16{"speed"}."speed" ("Enum") -> [w622]
        shift-right: [w621] -> _
        shift-left: w472 -> [w623]
        tunnel: w471 -> [w619]
        tunnel: w470 -> [w618]
        shift-right: [w614] -> _
        shift-left: w469 -> [w615]
        shift-right: [w613] -> _
        shift-left: enum16{"speed"}."speed" ("Enum") -> [w612]
        shift-right: [w611] -> _
        shift-left: w467 -> [w610]
        shift-left: w467 -> [w609]
        shift-right: [w608] -> _
        shift-left: w466 -> [w607]
        shift-left: w466 -> [w606]
        tunnel: w465 -> [w529]
        tunnel: w464 -> [w528]
        tunnel: [w588] -> w463
        tunnel: [w587] -> w462
        shift-right: [w553] -> _
        shift-left: w457 -> [w555]
        shift-left: w457 -> [w554]
        shift-right: [w550] -> _
        shift-left: w456 -> [w551]
        shift-left: w456 -> [w552]
        shift-right: [w549] -> _
        shift-left: w460 -> [w558]
        shift-right: [w548] -> _
        shift-left: enum16{"speed"}."speed" ("Enum") -> [w559]
        shift-right: [w547] -> _
        shift-left: w459 -> [w557]
        shift-right: [w546] -> _
        shift-left: enum16{"speed"}."speed" ("Enum") -> [w556]
        tunnel: [w529] -> w455
        tunnel: [w528] -> w454
        tunnel: [w525] -> w451
        tunnel: [w526] -> w452
        tunnel: [w527] -> w453
        shift-right: [w520] -> _
        shift-left: w449 -> [w522]
        shift-right: [w521] -> _
        shift-left: enum16{"speed"}."speed" ("Enum") -> [w523]
        shift-right: [w519] -> _
        shift-left: w445 -> [w518]
        shift-left: w445 -> [w517]
        shift-right: [w514] -> _
        shift-left: w448 -> [w516]
        shift-right: [w513] -> _
        shift-left: enum16{"speed"}."speed" ("Enum") -> [w515]
        shift-right: [w512] -> _
        shift-left: w446 -> [w511]
        shift-left: w446 -> [w510]
        tunnel: [w509] -> w442
        tunnel: w444 -> [w509]
        tunnel: [w508] -> w441
        tunnel: w443 -> [w508]
        tunnel: [w475] -> w440
        tunnel: [w474] -> w439
        stop <- w570 stop-if-true
        # "假終點"
        # "以下雙方向障礙"
        n277 = local read "遊玩時間"() -> (w568:i32)
        n278 = case shown="\"speed\"" w612 {
          tunnel: w615 -> [w838]
          tunnel: [w836] -> w614
          tunnel: [w835] -> w613
          tunnel: [w819] -> w611
          tunnel: w610 -> [w818]
          tunnel: w610 -> [w817]
          tunnel: w609 -> [w816]
          tunnel: w609 -> [w815]
          frame "speed" {
            n279 = Tick Count (ms)() -> (millisecond timer value=w847:u32)
            n280 = property on="X障礙" class="Bool (strict)"() -> ("Left"=w839:i32)  [unwired: 2 in, 2 out]
            n281 = property on="X障礙" class="Bool (strict)"() -> ("Left"=w833:i32)  [unwired: 2 in, 2 out]
            n282 = Less?(x=w833, y=0) -> (x < y?=w831:bool)
            n283 = Greater?(x=w818, y=500.0) -> (0:w813:bool)
            n284 = Greater?(x=w816, y=500.0) -> (0:w822:bool)
            n285 = Less?(x=w817, y=0.0) -> (x < y?=w825:bool)
            n286 = Less?(x=w815, y=0.0) -> (x < y?=w826:bool)
            n287 = Greater?(x=w839, y=500) -> (0:w830:bool)
            n288 = Subtract(x=w847, y=w838) -> (x-y=w846:u32)
            n289 = Or(x=w830, y=w831) -> (x .or. y?=w829:bool)
            n290 = To Double Precision Float(number=w846) -> (double precision float=w845:dbl)
            n291 = And(x=w813, y=w822) -> (x .and. y?=w827:bool)
            n292 = And(x=w825, y=w826) -> (x .and. y?=w828:bool)
            n293 = Or(x=w827, y=w828) -> (x .or. y?=w814:bool)
            n294 = local read "Vx"() -> (w834:i32)
            n295 = local read "x觸及位置"() -> (w841:i32)
            n296 = Divide(x=w845, y=1000.0) -> (x/y=w843:dbl)
            n297 = case shown="True" w814 {
              frame False {
              }
              frame True {
                w848 = 200 ("x觸及位置")
                n298 = local write "x觸及位置"(w848) -> ()
                n299 = Wait (ms)(milliseconds to wait=u32 100) -> ()  [unwired: 1 out]
                n300 = property on="X障礙" class="Bool (strict)"("Left"=w848) -> ()  [unwired: 2 in, 2 out]
              }
            }
            n301 = Multiply(x=w843, y=w834) -> (x*y=w842:dbl)
            n302 = Add(x=w842, y=w841) -> (x+y=w837:dbl)
            n303 = case shown="True" w829 {
              tunnel: [enum16{"speed"}."speed" ("Enum") enum16{"speed"}."speed" ("Enum")] -> w835
              tunnel: [w850 w857] -> w836
              tunnel: w838 -> [w850 _]
              tunnel: w837 -> [_ w853]
              tunnel: w834 -> [_ w855]
              frame False {
              }
              frame True {
                n304 = local write "x觸及位置"(w853) -> ()
                n305 = Multiply(x=w855, y=-1.0) -> (x*y=w852:dbl)
                n306 = Wait (ms)(milliseconds to wait=u32 25) -> ()  [unwired: 1 out]
                n307 = Tick Count (ms)() -> (millisecond timer value=w857:u32)
                n308 = local write "Vx"(w852) -> ()
              }
            }
            n309 = property on="X障礙" class="Bool (strict)"("Left"=w837) -> ()  [unwired: 2 in, 2 out]
            n310 = Wait (ms)(milliseconds to wait=u32 10) -> ()  [unwired: 1 out]
            n311 = property on="X障礙" class="Bool (strict)"() -> ("Left"=w819:i32)  [unwired: 2 in, 2 out]
          }
        }
        n312 = case shown="\"speed\"" w523 {
          tunnel: w522 -> [w697]
          tunnel: [w695] -> w520
          tunnel: [w694] -> w521
          tunnel: [w678] -> w519
          tunnel: w518 -> [w677]
          tunnel: w518 -> [w676]
          tunnel: w517 -> [w675]
          tunnel: w517 -> [w674]
          frame "speed" {
            n313 = Tick Count (ms)() -> (millisecond timer value=w706:u32)
            n314 = property on="Y障礙 2" class="Bool (strict)"() -> ("Top"=w698:i32)  [unwired: 2 in, 2 out]
            n315 = property on="Y障礙 2" class="Bool (strict)"() -> ("Top"=w692:i32)  [unwired: 2 in, 2 out]
            n316 = Less?(x=w692, y=0) -> (x < y?=w690:bool)
            n317 = Greater?(x=w677, y=400.0) -> (0:w672:bool)
            n318 = Greater?(x=w675, y=400.0) -> (0:w681:bool)
            n319 = Less?(x=w676, y=0.0) -> (x < y?=w684:bool)
            n320 = Less?(x=w674, y=0.0) -> (x < y?=w685:bool)
            n321 = Greater?(x=w698, y=400) -> (0:w689:bool)
            n322 = Subtract(x=w706, y=w697) -> (x-y=w705:u32)
            n323 = Or(x=w689, y=w690) -> (x .or. y?=w688:bool)
            n324 = To Double Precision Float(number=w705) -> (double precision float=w704:dbl)
            n325 = And(x=w672, y=w681) -> (x .and. y?=w686:bool)
            n326 = And(x=w684, y=w685) -> (x .and. y?=w687:bool)
            n327 = Or(x=w686, y=w687) -> (x .or. y?=w673:bool)
            n328 = local read "Vy 2"() -> (w693:i32)
            n329 = local read "y觸及位置 2"() -> (w700:i32)
            n330 = Divide(x=w704, y=1000.0) -> (x/y=w702:dbl)
            n331 = case shown="True" w673 {
              frame False {
              }
              frame True {
                w707 = 200 ("x觸及位置")
                n332 = local write "y觸及位置 2"(w707) -> ()
                n333 = Wait (ms)(milliseconds to wait=u32 100) -> ()  [unwired: 1 out]
                n334 = property on="Y障礙 2" class="Bool (strict)"("Top"=w707) -> ()  [unwired: 2 in, 2 out]
              }
            }
            n335 = Multiply(x=w702, y=w693) -> (x*y=w701:dbl)
            n336 = Add(x=w701, y=w700) -> (x+y=w696:dbl)
            n337 = case shown="True" w688 {
              tunnel: [enum16{"speed"}."speed" ("Enum") enum16{"speed"}."speed" ("Enum")] -> w694
              tunnel: [w709 w716] -> w695
              tunnel: w697 -> [w709 _]
              tunnel: w696 -> [_ w712]
              tunnel: w693 -> [_ w714]
              frame False {
              }
              frame True {
                n338 = local write "y觸及位置 2"(w712) -> ()
                n339 = Multiply(x=w714, y=-1.0) -> (x*y=w711:dbl)
                n340 = Wait (ms)(milliseconds to wait=u32 25) -> ()  [unwired: 1 out]
                n341 = local write "Vy 2"(w711) -> ()
                n342 = Tick Count (ms)() -> (millisecond timer value=w716:u32)
              }
            }
            n343 = property on="Y障礙 2" class="Bool (strict)"("Top"=w696) -> ()  [unwired: 2 in, 2 out]
            n344 = Wait (ms)(milliseconds to wait=u32 10) -> ()  [unwired: 1 out]
            n345 = property on="Y障礙 2" class="Bool (strict)"() -> ("Top"=w678:i32)  [unwired: 2 in, 2 out]
          }
        }
        n346 = case shown="\"speed\"" w559 {
          tunnel: w558 -> [w791]
          tunnel: [w789] -> w549
          tunnel: [w788] -> w548
          tunnel: [w772] -> w553
          tunnel: w555 -> [w771]
          tunnel: w555 -> [w770]
          tunnel: w554 -> [w769]
          tunnel: w554 -> [w768]
          frame "speed" {
            n347 = Tick Count (ms)() -> (millisecond timer value=w800:u32)
            n348 = property on="魔王" class="Bool (strict)"() -> ("Left"=w792:i32)  [unwired: 2 in, 2 out]
            n349 = property on="魔王" class="Bool (strict)"() -> ("Left"=w786:i32)  [unwired: 2 in, 2 out]
            n350 = Less?(x=w786, y=0) -> (x < y?=w784:bool)
            n351 = Greater?(x=w771, y=500.0) -> (0:w766:bool)
            n352 = Greater?(x=w769, y=500.0) -> (0:w775:bool)
            n353 = Less?(x=w770, y=0.0) -> (x < y?=w778:bool)
            n354 = Less?(x=w768, y=0.0) -> (x < y?=w779:bool)
            n355 = Greater?(x=w792, y=500) -> (0:w783:bool)
            n356 = Subtract(x=w800, y=w791) -> (x-y=w799:u32)
            n357 = Or(x=w783, y=w784) -> (x .or. y?=w782:bool)
            n358 = To Double Precision Float(number=w799) -> (double precision float=w798:dbl)
            n359 = And(x=w766, y=w775) -> (x .and. y?=w780:bool)
            n360 = And(x=w778, y=w779) -> (x .and. y?=w781:bool)
            n361 = Or(x=w780, y=w781) -> (x .or. y?=w767:bool)
            n362 = local read "Å]Vx"() -> (w787:i32)
            n363 = Divide(x=w798, y=1000.0) -> (x/y=w796:dbl)
            n364 = local read "Å]XÄ²"() -> (w794:i32)
            n365 = case shown="True" w767 {
              frame False {
              }
              frame True {
                w801 = 200 ("x觸及位置")
                n366 = local write "Å]XÄ²"(w801) -> ()
                n367 = Wait (ms)(milliseconds to wait=u32 100) -> ()  [unwired: 1 out]
                n368 = property on="魔王" class="Bool (strict)"("Left"=w801) -> ()  [unwired: 2 in, 2 out]
              }
            }
            n369 = Multiply(x=w796, y=w787) -> (x*y=w795:dbl)
            n370 = Add(x=w795, y=w794) -> (x+y=w790:dbl)
            n371 = case shown="True" w782 {
              tunnel: [enum16{"speed"}."speed" ("Enum") enum16{"speed"}."speed" ("Enum")] -> w788
              tunnel: [w803 w810] -> w789
              tunnel: w791 -> [w803 _]
              tunnel: w790 -> [_ w806]
              tunnel: w787 -> [_ w808]
              frame False {
              }
              frame True {
                n372 = Multiply(x=w808, y=-1.0) -> (x*y=w805:dbl)
                n373 = local write "Å]XÄ²"(w806) -> ()
                n374 = Wait (ms)(milliseconds to wait=u32 25) -> ()  [unwired: 1 out]
                n375 = local write "Å]Vx"(w805) -> ()
                n376 = Tick Count (ms)() -> (millisecond timer value=w810:u32)
              }
            }
            n377 = property on="魔王" class="Bool (strict)"("Left"=w790) -> ()  [unwired: 2 in, 2 out]
            n378 = Wait (ms)(milliseconds to wait=u32 10) -> ()  [unwired: 1 out]
            n379 = property on="魔王" class="Bool (strict)"() -> ("Left"=w772:i32)  [unwired: 2 in, 2 out]
          }
        }
        n380 = case shown="\"speed\"" w556 {
          tunnel: w557 -> [w744]
          tunnel: [w742] -> w547
          tunnel: [w741] -> w546
          tunnel: [w725] -> w550
          tunnel: w552 -> [w724]
          tunnel: w552 -> [w723]
          tunnel: w551 -> [w722]
          tunnel: w551 -> [w721]
          frame "speed" {
            n381 = Tick Count (ms)() -> (millisecond timer value=w753:u32)
            n382 = property on="魔王" class="Bool (strict)"() -> ("Top"=w745:i32)  [unwired: 2 in, 2 out]
            n383 = property on="魔王" class="Bool (strict)"() -> ("Top"=w739:i32)  [unwired: 2 in, 2 out]
            n384 = Less?(x=w739, y=0) -> (x < y?=w737:bool)
            n385 = Greater?(x=w724, y=400.0) -> (0:w719:bool)
            n386 = Greater?(x=w722, y=400.0) -> (0:w728:bool)
            n387 = Less?(x=w723, y=0.0) -> (x < y?=w731:bool)
            n388 = Less?(x=w721, y=0.0) -> (x < y?=w732:bool)
            n389 = Greater?(x=w745, y=400) -> (0:w736:bool)
            n390 = Subtract(x=w753, y=w744) -> (x-y=w752:u32)
            n391 = Or(x=w736, y=w737) -> (x .or. y?=w735:bool)
            n392 = To Double Precision Float(number=w752) -> (double precision float=w751:dbl)
            n393 = And(x=w719, y=w728) -> (x .and. y?=w733:bool)
            n394 = And(x=w731, y=w732) -> (x .and. y?=w734:bool)
            n395 = Or(x=w733, y=w734) -> (x .or. y?=w720:bool)
            n396 = local read "Å]Vy"() -> (w740:i64)
            n397 = Divide(x=w751, y=1000.0) -> (x/y=w749:dbl)
            n398 = local read "Å]YÄ²"() -> (w747:i32)
            n399 = case shown="True" w720 {
              frame False {
              }
              frame True {
                w754 = 200 ("x觸及位置")
                n400 = local write "Å]YÄ²"(w754) -> ()
                n401 = Wait (ms)(milliseconds to wait=u32 100) -> ()  [unwired: 1 out]
                n402 = property on="魔王" class="Bool (strict)"("Top"=w754) -> ()  [unwired: 2 in, 2 out]
              }
            }
            n403 = Multiply(x=w749, y=w740) -> (x*y=w748:dbl)
            n404 = Add(x=w748, y=w747) -> (x+y=w743:dbl)
            n405 = case shown="True" w735 {
              tunnel: [enum16{"speed"}."speed" ("Enum") enum16{"speed"}."speed" ("Enum")] -> w741
              tunnel: [w756 w763] -> w742
              tunnel: w744 -> [w756 _]
              tunnel: w743 -> [_ w759]
              tunnel: w740 -> [_ w761]
              frame False {
              }
              frame True {
                n406 = Multiply(x=w761, y=-1.0) -> (x*y=w758:dbl)
                n407 = local write "Å]YÄ²"(w759) -> ()
                n408 = Wait (ms)(milliseconds to wait=u32 25) -> ()  [unwired: 1 out]
                n409 = local write "Å]Vy"(w758) -> ()
                n410 = Tick Count (ms)() -> (millisecond timer value=w763:u32)
              }
            }
            n411 = property on="魔王" class="Bool (strict)"("Top"=w743) -> ()  [unwired: 2 in, 2 out]
            n412 = Wait (ms)(milliseconds to wait=u32 10) -> ()  [unwired: 1 out]
            n413 = property on="魔王" class="Bool (strict)"() -> ("Top"=w725:i32)  [unwired: 2 in, 2 out]
          }
        }
        n414 = case shown="\"speed\"" w515 {
          tunnel: w516 -> [w650]
          tunnel: [w648] -> w514
          tunnel: [w647] -> w513
          tunnel: [w631] -> w512
          tunnel: w511 -> [w630]
          tunnel: w511 -> [w629]
          tunnel: w510 -> [w628]
          tunnel: w510 -> [w627]
          frame "speed" {
            n415 = Tick Count (ms)() -> (millisecond timer value=w659:u32)
            n416 = property on="X障礙 2" class="Bool (strict)"() -> ("Left"=w651:i32)  [unwired: 2 in, 2 out]
            n417 = property on="X障礙 2" class="Bool (strict)"() -> ("Left"=w645:i32)  [unwired: 2 in, 2 out]
            n418 = Less?(x=w645, y=0) -> (x < y?=w643:bool)
            n419 = Greater?(x=w630, y=500.0) -> (0:w625:bool)
            n420 = Greater?(x=w628, y=500.0) -> (0:w634:bool)
            n421 = Less?(x=w629, y=0.0) -> (x < y?=w637:bool)
            n422 = Less?(x=w627, y=0.0) -> (x < y?=w638:bool)
            n423 = Greater?(x=w651, y=500) -> (0:w642:bool)
            n424 = Subtract(x=w659, y=w650) -> (x-y=w658:u32)
            n425 = Or(x=w642, y=w643) -> (x .or. y?=w641:bool)
            n426 = To Double Precision Float(number=w658) -> (double precision float=w657:dbl)
            n427 = And(x=w625, y=w634) -> (x .and. y?=w639:bool)
            n428 = And(x=w637, y=w638) -> (x .and. y?=w640:bool)
            n429 = Or(x=w639, y=w640) -> (x .or. y?=w626:bool)
            n430 = local read "Vx 2"() -> (w646:i32)
            n431 = local read "x觸及位置 2"() -> (w653:i32)
            n432 = Divide(x=w657, y=1000.0) -> (x/y=w655:dbl)
            n433 = case shown="True" w626 {
              frame False {
              }
              frame True {
                w660 = 200 ("x觸及位置")
                n434 = local write "x觸及位置 2"(w660) -> ()
                n435 = Wait (ms)(milliseconds to wait=u32 100) -> ()  [unwired: 1 out]
                n436 = property on="X障礙 2" class="Bool (strict)"("Left"=w660) -> ()  [unwired: 2 in, 2 out]
              }
            }
            n437 = Multiply(x=w655, y=w646) -> (x*y=w654:dbl)
            n438 = Add(x=w654, y=w653) -> (x+y=w649:dbl)
            n439 = case shown="True" w641 {
              tunnel: [enum16{"speed"}."speed" ("Enum") enum16{"speed"}."speed" ("Enum")] -> w647
              tunnel: [w662 w669] -> w648
              tunnel: w650 -> [w662 _]
              tunnel: w649 -> [_ w665]
              tunnel: w646 -> [_ w667]
              frame False {
              }
              frame True {
                n440 = local write "x觸及位置 2"(w665) -> ()
                n441 = Multiply(x=w667, y=-1.0) -> (x*y=w664:dbl)
                n442 = Wait (ms)(milliseconds to wait=u32 25) -> ()  [unwired: 1 out]
                n443 = local write "Vx 2"(w664) -> ()
                n444 = Tick Count (ms)() -> (millisecond timer value=w669:u32)
              }
            }
            n445 = property on="X障礙 2" class="Bool (strict)"("Left"=w649) -> ()  [unwired: 2 in, 2 out]
            n446 = Wait (ms)(milliseconds to wait=u32 10) -> ()  [unwired: 1 out]
            n447 = property on="X障礙 2" class="Bool (strict)"() -> ("Left"=w631:i32)  [unwired: 2 in, 2 out]
          }
        }
        n448 = case shown="\"speed\"" w622 {
          tunnel: w623 -> [w901]
          tunnel: [w899] -> w621
          tunnel: [w898] -> w620
          tunnel: [w882] -> w608
          tunnel: w607 -> [w881]
          tunnel: w607 -> [w880]
          tunnel: w606 -> [w879]
          tunnel: w606 -> [w878]
          frame "speed" {
            n449 = Tick Count (ms)() -> (millisecond timer value=w910:u32)
            n450 = Greater?(x=w881, y=400.0) -> (0:w876:bool)
            n451 = Greater?(x=w879, y=400.0) -> (0:w885:bool)
            n452 = Less?(x=w880, y=0.0) -> (x < y?=w888:bool)
            n453 = Less?(x=w878, y=0.0) -> (x < y?=w889:bool)
            n454 = property on="Y障礙" class="Bool (strict)"() -> ("Top"=w902:i32)  [unwired: 2 in, 2 out]
            n455 = property on="Y障礙" class="Bool (strict)"() -> ("Top"=w896:i32)  [unwired: 2 in, 2 out]
            n456 = Less?(x=w896, y=0) -> (x < y?=w894:bool)
            n457 = Greater?(x=w902, y=400) -> (0:w893:bool)
            n458 = Subtract(x=w910, y=w901) -> (x-y=w909:u32)
            n459 = Or(x=w893, y=w894) -> (x .or. y?=w892:bool)
            n460 = And(x=w876, y=w885) -> (x .and. y?=w890:bool)
            n461 = And(x=w888, y=w889) -> (x .and. y?=w891:bool)
            n462 = To Double Precision Float(number=w909) -> (double precision float=w908:dbl)
            n463 = Or(x=w890, y=w891) -> (x .or. y?=w877:bool)
            n464 = local read "Vy"() -> (w897:i32)
            n465 = local read "y觸及位置"() -> (w904:i32)
            n466 = Divide(x=w908, y=1000.0) -> (x/y=w906:dbl)
            n467 = case shown="True" w877 {
              frame False {
              }
              frame True {
                w911 = 200 ("y觸及位置")
                n468 = local write "y觸及位置"(w911) -> ()
                n469 = Wait (ms)(milliseconds to wait=u32 100) -> ()  [unwired: 1 out]
                n470 = property on="Y障礙" class="Bool (strict)"("Top"=w911) -> ()  [unwired: 2 in, 2 out]
              }
            }
            n471 = Multiply(x=w906, y=w897) -> (x*y=w905:dbl)
            n472 = Add(x=w905, y=w904) -> (x+y=w900:dbl)
            n473 = case shown="True" w892 {
              tunnel: [enum16{"speed"}."speed" ("Enum") enum16{"speed"}."speed" ("Enum")] -> w898
              tunnel: [w913 w920] -> w899
              tunnel: w901 -> [w913 _]
              tunnel: w900 -> [_ w916]
              tunnel: w897 -> [_ w918]
              frame False {
              }
              frame True {
                n474 = local write "y觸及位置"(w916) -> ()
                n475 = Multiply(x=w918, y=-1.0) -> (x*y=w915:dbl)
                n476 = Wait (ms)(milliseconds to wait=u32 25) -> ()  [unwired: 1 out]
                n477 = Tick Count (ms)() -> (millisecond timer value=w920:u32)
                n478 = local write "Vy"(w915) -> ()
              }
            }
            n479 = property on="Y障礙" class="Bool (strict)"("Top"=w900) -> ()  [unwired: 2 in, 2 out]
            n480 = property on="Y障礙" class="Bool (strict)"() -> ("Top"=w882:i32)  [unwired: 2 in, 2 out]
            n481 = Wait (ms)(milliseconds to wait=u32 10) -> ()  [unwired: 1 out]
          }
        }
        n482 = call-poly <vilib>:"Acquire Input Data.vi"("device ID"=w619, "error in (no error)"=w618) -> ("device ID"=w588:refnum<k1>, "keys pressed"=w617:T1, "error out"=w587:errorcluster)  [unwired: 15 in]
        n483 = Increment(x=w568) -> (x+1=w569:i32)
        n484 = local write "遊玩時間"(w569) -> ()
        n485 = Array To Cluster(array=w617) -> (cluster=w605:T2)
        n486 = Unbundle(w605) -> ("keys pressed[0]"=w616:T3)  [unwired: 8 out]
        n487 = case shown="\"A\"" w616 {
          frame Default {
          }
          frame "A" {
            n488 = local read "X"() -> (w873:dbl)
            n489 = Wait (ms)(milliseconds to wait=u32 10) -> ()  [unwired: 1 out]
            n490 = Add(x=-2.0, y=w873) -> (x+y=w871:dbl)
            n491 = local write "X"(w871) -> ()
            n492 = property on="小精靈" class="Bool (strict)"("Left"=w871) -> ()  [unwired: 2 in, 2 out]
          }
        }
        n493 = case shown="\"D\"" w616 {
          frame Default {
          }
          frame "D" {
            n494 = local read "X"() -> (w869:dbl)
            n495 = Wait (ms)(milliseconds to wait=u32 10) -> ()  [unwired: 1 out]
            n496 = Add(x=2.0, y=w869) -> (x+y=w867:dbl)
            n497 = local write "X"(w867) -> ()
            n498 = property on="小精靈" class="Bool (strict)"("Left"=w867) -> ()  [unwired: 2 in, 2 out]
          }
        }
        n499 = property on="Y障礙" class="Bool (strict)"() -> ("Top"=w589:i32)  [unwired: 2 in, 2 out]
        n500 = property on="Y障礙" class="Bool (strict)"() -> ("Top"=w595:i32)  [unwired: 2 in, 2 out]
        n501 = property on="Y障礙" class="Bool (strict)"() -> ("Left"=w602:i32)  [unwired: 2 in, 2 out]
        n502 = property on="Y障礙" class="Bool (strict)"() -> ("Left"=w600:i32)  [unwired: 2 in, 2 out]
        n503 = case shown="\"W\"" w616 {
          frame Default {
          }
          frame "W" {
            n504 = local read "Y"() -> (w865:dbl)
            n505 = Wait (ms)(milliseconds to wait=u32 10) -> ()  [unwired: 1 out]
            n506 = Add(x=-2.0, y=w865) -> (x+y=w863:dbl)
            n507 = local write "Y"(w863) -> ()
            n508 = property on="小精靈" class="Bool (strict)"("Top"=w863) -> ()  [unwired: 2 in, 2 out]
          }
        }
        n509 = case shown="\"S\"" w616 {
          frame Default {
          }
          frame "S" {
            n510 = local read "Y"() -> (w861:dbl)
            n511 = Wait (ms)(milliseconds to wait=u32 10) -> ()  [unwired: 1 out]
            n512 = Add(x=2.0, y=w861) -> (x+y=w859:dbl)
            n513 = local write "Y"(w859) -> ()
            n514 = property on="小精靈" class="Bool (strict)"("Top"=w859) -> ()  [unwired: 2 in, 2 out]
          }
        }
        n515 = local read "Y"() -> (w603:dbl)
        n516 = local read "X"() -> (w604:dbl)
        n517 = Add(x=w602, y=17) -> (x+y=w597:i32)
        n518 = Subtract(x=w600, y=17) -> (x-y=w598:i32)
        n519 = Subtract(x=w595, y=15) -> (x-y=w594:i32)
        n520 = Add(x=w589, y=20) -> (x+y=w590:i32)
        n521 = In Range and Coerce(upper limit=w597, x=w604, lower limit=w598) -> (In Range?=w593:bool)  [unwired: 1 out]
        n522 = In Range and Coerce(upper limit=w590, x=w603, lower limit=w594) -> (In Range?=w592:bool)  [unwired: 1 out]
        n523 = And(x=w593, y=w592) -> (x .and. y?=w527:bool)
        n524 = property on="X障礙" class="Bool (strict)"() -> ("Top"=w586:i32)  [unwired: 2 in, 2 out]
        n525 = property on="X障礙" class="Bool (strict)"() -> ("Top"=w580:i32)  [unwired: 2 in, 2 out]
        n526 = property on="X障礙" class="Bool (strict)"() -> ("Left"=w573:i32)  [unwired: 2 in, 2 out]
        n527 = property on="X障礙" class="Bool (strict)"() -> ("Left"=w575:i32)  [unwired: 2 in, 2 out]
        n528 = local read "Y"() -> (w572:dbl)
        n529 = property on="魔王" class="Bool (strict)"() -> ("Top"=w530:i32)  [unwired: 2 in, 2 out]
        n530 = property on="魔王" class="Bool (strict)"() -> ("Top"=w536:i32)  [unwired: 2 in, 2 out]
        n531 = property on="魔王" class="Bool (strict)"() -> ("Left"=w543:i32)  [unwired: 2 in, 2 out]
        n532 = property on="魔王" class="Bool (strict)"() -> ("Left"=w541:i32)  [unwired: 2 in, 2 out]
        n533 = local read "X"() -> (w571:dbl)
        n534 = local read "X"() -> (w567:dbl)
        n535 = local read "Y"() -> (w566:dbl)
        n536 = property on="X障礙 2" class="Bool (strict)"() -> ("Top"=w507:i32)  [unwired: 2 in, 2 out]
        n537 = property on="X障礙 2" class="Bool (strict)"() -> ("Top"=w501:i32)  [unwired: 2 in, 2 out]
        n538 = property on="X障礙 2" class="Bool (strict)"() -> ("Left"=w494:i32)  [unwired: 2 in, 2 out]
        n539 = property on="X障礙 2" class="Bool (strict)"() -> ("Left"=w496:i32)  [unwired: 2 in, 2 out]
        n540 = property on="Y障礙 2" class="Bool (strict)"() -> ("Top"=w491:i32)  [unwired: 2 in, 2 out]
        n541 = property on="Y障礙 2" class="Bool (strict)"() -> ("Top"=w485:i32)  [unwired: 2 in, 2 out]
        n542 = property on="Y障礙 2" class="Bool (strict)"() -> ("Left"=w478:i32)  [unwired: 2 in, 2 out]
        n543 = property on="Y障礙 2" class="Bool (strict)"() -> ("Left"=w480:i32)  [unwired: 2 in, 2 out]
        n544 = local read "Y"() -> (w544:dbl)
        n545 = local read "X"() -> (w545:dbl)
        n546 = local read "Y"() -> (w493:dbl)
        n547 = local read "Y"() -> (w477:dbl)
        n548 = Add(x=w573, y=17) -> (x+y=w578:i32)
        n549 = Subtract(x=w575, y=17) -> (x-y=w577:i32)
        n550 = Subtract(x=w580, y=15) -> (x-y=w581:i32)
        n551 = local read "X"() -> (w492:dbl)
        n552 = local read "X"() -> (w476:dbl)
        n553 = Add(x=w586, y=20) -> (x+y=w585:i32)
        n554 = In Range and Coerce(upper limit=516.0, x=w567, lower limit=463.0) -> (In Range?=w565:bool)  [unwired: 1 out]
        n555 = In Range and Coerce(upper limit=399.0, x=w566, lower limit=358.0) -> (In Range?=w564:bool)  [unwired: 1 out]
        n556 = Add(x=w543, y=17) -> (x+y=w538:i32)
        n557 = Subtract(x=w541, y=17) -> (x-y=w539:i32)
        n558 = Subtract(x=w536, y=15) -> (x-y=w535:i32)
        n559 = Add(x=w530, y=20) -> (x+y=w531:i32)
        n560 = Add(x=w494, y=17) -> (x+y=w499:i32)
        n561 = Subtract(x=w496, y=17) -> (x-y=w498:i32)
        n562 = Subtract(x=w501, y=15) -> (x-y=w502:i32)
        n563 = Add(x=w478, y=17) -> (x+y=w483:i32)
        n564 = Subtract(x=w480, y=17) -> (x-y=w482:i32)
        n565 = Subtract(x=w485, y=15) -> (x-y=w486:i32)
        n566 = In Range and Coerce(upper limit=w578, x=w571, lower limit=w577) -> (In Range?=w582:bool)  [unwired: 1 out]
        n567 = In Range and Coerce(upper limit=w585, x=w572, lower limit=w581) -> (In Range?=w583:bool)  [unwired: 1 out]
        n568 = Add(x=w507, y=20) -> (x+y=w506:i32)
        n569 = Add(x=w491, y=20) -> (x+y=w490:i32)
        n570 = And(x=w565, y=w564) -> (x .and. y?=w524:bool)
        n571 = In Range and Coerce(upper limit=w538, x=w545, lower limit=w539) -> (In Range?=w534:bool)  [unwired: 1 out]
        n572 = In Range and Coerce(upper limit=w531, x=w544, lower limit=w535) -> (In Range?=w533:bool)  [unwired: 1 out]
        n573 = And(x=w582, y=w583) -> (x .and. y?=w526:bool)
        n574 = In Range and Coerce(upper limit=w499, x=w492, lower limit=w498) -> (In Range?=w503:bool)  [unwired: 1 out]
        n575 = In Range and Coerce(upper limit=w506, x=w493, lower limit=w502) -> (In Range?=w504:bool)  [unwired: 1 out]
        n576 = In Range and Coerce(upper limit=w483, x=w476, lower limit=w482) -> (In Range?=w487:bool)  [unwired: 1 out]
        n577 = In Range and Coerce(upper limit=w490, x=w477, lower limit=w486) -> (In Range?=w488:bool)  [unwired: 1 out]
        n578 = And(x=w534, y=w533) -> (x .and. y?=w525:bool)
        n579 = And(x=w503, y=w504) -> (x .and. y?=w475:bool)
        n580 = And(x=w487, y=w488) -> (x .and. y?=w474:bool)
        n581 = Compound Arithmetic op=OR(w474, w475, w508, w509, w529, w528, w527, w526, w525, w524) -> (w570:bool)
      }
      n582 = call-poly <vilib>:"Close Input Device.vi"("error in (no error)"=w462, "device ID"=w463) -> ()  [unwired: 8 in, 1 out]
    }
    frame #4 {
      w934 = 0 ("Position:Left")
      w935 = 1 ("Position:Left")
      n583 = property on="Y障礙 2" class="Bool (strict)"("Left"=80 ("Position:Left"), "Top"=1 ("Position:Top")) -> ()  [unwired: 2 in, 2 out]
      n584 = property on="Y障礙" class="Bool (strict)"("Left"=375 ("Position:Left"), "Top"=1 ("Position:Top")) -> ()  [unwired: 2 in, 2 out]
      n585 = local write "x觸及位置 2"(0 ("x觸及位置")) -> ()
      n586 = property on="魔王" class="Bool (strict)"("Left"=w935, "Top"=w935) -> ()  [unwired: 2 in, 2 out]
      n587 = local write "y觸及位置 2"(0 ("y觸及位置")) -> ()
      n588 = local write "Vy"(400 ("Vy")) -> ()
      n589 = local write "Vx"(400 ("Vx")) -> ()
      n590 = local write "y觸及位置"(0 ("y觸及位置")) -> ()
      n591 = local write "x觸及位置"(0 ("x觸及位置")) -> ()
      n592 = local write "Å]XÄ²"(0 ("Vy")) -> ()
      n593 = local write "Å]Vx"(500 ("Vy")) -> ()
      n594 = local write "Å]Vy"(500 ("Vx")) -> ()
      n595 = local write "Å]YÄ²"(0 ("Vx")) -> ()
      n596 = property on="X障礙 2" class="Bool (strict)"("Left"=1 ("Position:Left"), "Top"=60 ("Position:Top")) -> ()  [unwired: 2 in, 2 out]
      n597 = local write "Vx 2"(350 ("Vx 2")) -> ()
      n598 = property on="X障礙" class="Bool (strict)"("Left"=1 ("Position:Left"), "Top"=340 ("Position:Top")) -> ()  [unwired: 2 in, 2 out]
      n599 = local write "Vy 2"(350 ("Vy 2")) -> ()
      n600 = property on="終點" class="Bool (strict)"("Left"=w934, "Top"=w934) -> ()  [unwired: 2 in, 2 out]
    }
    frame #5 {
      w953 = 0 ("Left")
      w956 = 0 ("Top")
      w963 = 0 ("Top")
      w968 = 0 ("Left")
      w964 = 0 ("Left")
      w975 = 0 ("Top")
      n601 = Tick Count (ms)() -> (millisecond timer value=w971:u32)
      n602 = Tick Count (ms)() -> (millisecond timer value=w966:u32)
      n603 = Tick Count (ms)() -> (millisecond timer value=w955:u32)
      n604 = Tick Count (ms)() -> (millisecond timer value=w969:u32)
      n605 = Tick Count (ms)() -> (millisecond timer value=w958:u32)
      n606 = call <vilib>:"Intialize Keyboard.vi"() -> ("error out"=w978:errorcluster, "device ID"=w979:refnum<k1>)  [unwired: 10 in]
      n607 = Tick Count (ms)() -> (millisecond timer value=w974:u32)
      n608 = while {
        shift-right: [w1136] -> _
        shift-left: enum16{"speed"}."speed" ("Enum") -> [w1138]
        shift-right: [w1137] -> _
        shift-left: w974 -> [w1139]
        tunnel: w979 -> [w1135]
        tunnel: w978 -> [w1134]
        shift-right: [w1130] -> _
        shift-left: w971 -> [w1131]
        shift-right: [w1129] -> _
        shift-left: enum16{"speed"}."speed" ("Enum") -> [w1128]
        shift-right: [w1127] -> _
        shift-left: w975 -> [w1126]
        shift-left: w975 -> [w1125]
        tunnel: [w1107] -> w977
        tunnel: [w1106] -> w976
        tunnel: [w1043] -> w965
        shift-right: [w1072] -> _
        shift-left: w968 -> [w1074]
        shift-left: w968 -> [w1073]
        shift-right: [w1071] -> _
        shift-left: w969 -> [w1077]
        shift-right: [w1070] -> _
        shift-left: enum16{"speed"}."speed" ("Enum") -> [w1078]
        shift-right: [w1069] -> _
        shift-left: w966 -> [w1076]
        shift-right: [w1068] -> _
        shift-left: enum16{"speed"}."speed" ("Enum") -> [w1075]
        tunnel: w984 -> [w1051]
        tunnel: w983 -> [w1050]
        tunnel: w982 -> [w1049]
        tunnel: w981 -> [w1048]
        tunnel: w980 -> [w1047]
        shift-right: [w1040] -> _
        shift-left: w964 -> [w1042]
        shift-left: w964 -> [w1041]
        shift-right: [w1037] -> _
        shift-left: w963 -> [w1039]
        shift-left: w963 -> [w1038]
        tunnel: w962 -> [w1036]
        tunnel: w961 -> [w1035]
        tunnel: w960 -> [w1034]
        tunnel: w959 -> [w1033]
        shift-right: [w1030] -> _
        shift-left: w958 -> [w1032]
        shift-right: [w1029] -> _
        shift-left: enum16{"speed"}."speed" ("Enum") -> [w1031]
        shift-right: [w1028] -> _
        shift-left: w956 -> [w1027]
        shift-left: w956 -> [w1026]
        shift-right: [w1023] -> _
        shift-left: w955 -> [w1025]
        shift-right: [w1022] -> _
        shift-left: enum16{"speed"}."speed" ("Enum") -> [w1024]
        shift-right: [w1021] -> _
        shift-left: w953 -> [w1020]
        shift-left: w953 -> [w1019]
        stop <- w1089 stop-if-true
        # "終點"
        # "以下雙方向障礙"
        n609 = local read "遊玩時間"() -> (w1087:i32)
        n610 = case shown="\"speed\"" w1128 {
          tunnel: w1131 -> [w1354]
          tunnel: [w1352] -> w1130
          tunnel: [w1351] -> w1129
          tunnel: [w1335] -> w1040
          tunnel: w1042 -> [w1334]
          tunnel: w1042 -> [w1333]
          tunnel: w1041 -> [w1332]
          tunnel: w1041 -> [w1331]
          frame "speed" {
            n611 = Tick Count (ms)() -> (millisecond timer value=w1363:u32)
            n612 = property on="X障礙" class="Bool (strict)"() -> ("Left"=w1355:i32)  [unwired: 2 in, 2 out]
            n613 = property on="X障礙" class="Bool (strict)"() -> ("Left"=w1349:i32)  [unwired: 2 in, 2 out]
            n614 = Less?(x=w1349, y=0) -> (x < y?=w1347:bool)
            n615 = Greater?(x=w1334, y=500.0) -> (0:w1329:bool)
            n616 = Greater?(x=w1332, y=500.0) -> (0:w1338:bool)
            n617 = Less?(x=w1333, y=0.0) -> (x < y?=w1341:bool)
            n618 = Less?(x=w1331, y=0.0) -> (x < y?=w1342:bool)
            n619 = Greater?(x=w1355, y=500) -> (0:w1346:bool)
            n620 = Subtract(x=w1363, y=w1354) -> (x-y=w1362:u32)
            n621 = Or(x=w1346, y=w1347) -> (x .or. y?=w1345:bool)
            n622 = To Double Precision Float(number=w1362) -> (double precision float=w1361:dbl)
            n623 = And(x=w1329, y=w1338) -> (x .and. y?=w1343:bool)
            n624 = And(x=w1341, y=w1342) -> (x .and. y?=w1344:bool)
            n625 = Or(x=w1343, y=w1344) -> (x .or. y?=w1330:bool)
            n626 = local read "Vx"() -> (w1350:i32)
            n627 = local read "x觸及位置"() -> (w1357:i32)
            n628 = Divide(x=w1361, y=1000.0) -> (x/y=w1359:dbl)
            n629 = case shown="True" w1330 {
              frame False {
              }
              frame True {
                w1364 = 200 ("x觸及位置")
                n630 = local write "x觸及位置"(w1364) -> ()
                n631 = Wait (ms)(milliseconds to wait=u32 100) -> ()  [unwired: 1 out]
                n632 = property on="X障礙" class="Bool (strict)"("Left"=w1364) -> ()  [unwired: 2 in, 2 out]
              }
            }
            n633 = Multiply(x=w1359, y=w1350) -> (x*y=w1358:dbl)
            n634 = Add(x=w1358, y=w1357) -> (x+y=w1353:dbl)
            n635 = case shown="True" w1345 {
              tunnel: [enum16{"speed"}."speed" ("Enum") enum16{"speed"}."speed" ("Enum")] -> w1351
              tunnel: [w1366 w1373] -> w1352
              tunnel: w1354 -> [w1366 _]
              tunnel: w1353 -> [_ w1369]
              tunnel: w1350 -> [_ w1371]
              frame False {
              }
              frame True {
                n636 = local write "x觸及位置"(w1369) -> ()
                n637 = Multiply(x=w1371, y=-1.0) -> (x*y=w1368:dbl)
                n638 = Wait (ms)(milliseconds to wait=u32 25) -> ()  [unwired: 1 out]
                n639 = Tick Count (ms)() -> (millisecond timer value=w1373:u32)
                n640 = local write "Vx"(w1368) -> ()
              }
            }
            n641 = property on="X障礙" class="Bool (strict)"("Left"=w1353) -> ()  [unwired: 2 in, 2 out]
            n642 = Wait (ms)(milliseconds to wait=u32 10) -> ()  [unwired: 1 out]
            n643 = property on="X障礙" class="Bool (strict)"() -> ("Left"=w1335:i32)  [unwired: 2 in, 2 out]
          }
        }
        n644 = case shown="\"speed\"" w1078 {
          tunnel: w1077 -> [w1307]
          tunnel: [w1305] -> w1071
          tunnel: [w1304] -> w1070
          tunnel: [w1288] -> w1072
          tunnel: w1074 -> [w1287]
          tunnel: w1074 -> [w1286]
          tunnel: w1073 -> [w1285]
          tunnel: w1073 -> [w1284]
          frame "speed" {
            n645 = Tick Count (ms)() -> (millisecond timer value=w1316:u32)
            n646 = property on="魔王" class="Bool (strict)"() -> ("Left"=w1308:i32)  [unwired: 2 in, 2 out]
            n647 = property on="魔王" class="Bool (strict)"() -> ("Left"=w1302:i32)  [unwired: 2 in, 2 out]
            n648 = Less?(x=w1302, y=0) -> (x < y?=w1300:bool)
            n649 = Greater?(x=w1287, y=500.0) -> (0:w1282:bool)
            n650 = Greater?(x=w1285, y=500.0) -> (0:w1291:bool)
            n651 = Less?(x=w1286, y=0.0) -> (x < y?=w1294:bool)
            n652 = Less?(x=w1284, y=0.0) -> (x < y?=w1295:bool)
            n653 = Greater?(x=w1308, y=500) -> (0:w1299:bool)
            n654 = Subtract(x=w1316, y=w1307) -> (x-y=w1315:u32)
            n655 = Or(x=w1299, y=w1300) -> (x .or. y?=w1298:bool)
            n656 = To Double Precision Float(number=w1315) -> (double precision float=w1314:dbl)
            n657 = And(x=w1282, y=w1291) -> (x .and. y?=w1296:bool)
            n658 = And(x=w1294, y=w1295) -> (x .and. y?=w1297:bool)
            n659 = Or(x=w1296, y=w1297) -> (x .or. y?=w1283:bool)
            n660 = local read "Å]Vx"() -> (w1303:i32)
            n661 = Divide(x=w1314, y=1000.0) -> (x/y=w1312:dbl)
            n662 = local read "Å]XÄ²"() -> (w1310:i32)
            n663 = case shown="True" w1283 {
              frame False {
              }
              frame True {
                w1317 = 200 ("x觸及位置")
                n664 = local write "Å]XÄ²"(w1317) -> ()
                n665 = Wait (ms)(milliseconds to wait=u32 100) -> ()  [unwired: 1 out]
                n666 = property on="魔王" class="Bool (strict)"("Left"=w1317) -> ()  [unwired: 2 in, 2 out]
              }
            }
            n667 = Multiply(x=w1312, y=w1303) -> (x*y=w1311:dbl)
            n668 = Add(x=w1311, y=w1310) -> (x+y=w1306:dbl)
            n669 = case shown="True" w1298 {
              tunnel: [enum16{"speed"}."speed" ("Enum") enum16{"speed"}."speed" ("Enum")] -> w1304
              tunnel: [w1319 w1326] -> w1305
              tunnel: w1307 -> [w1319 _]
              tunnel: w1306 -> [_ w1322]
              tunnel: w1303 -> [_ w1324]
              frame False {
              }
              frame True {
                n670 = Multiply(x=w1324, y=-1.0) -> (x*y=w1321:dbl)
                n671 = local write "Å]XÄ²"(w1322) -> ()
                n672 = Wait (ms)(milliseconds to wait=u32 25) -> ()  [unwired: 1 out]
                n673 = local write "Å]Vx"(w1321) -> ()
                n674 = Tick Count (ms)() -> (millisecond timer value=w1326:u32)
              }
            }
            n675 = property on="魔王" class="Bool (strict)"("Left"=w1306) -> ()  [unwired: 2 in, 2 out]
            n676 = Wait (ms)(milliseconds to wait=u32 10) -> ()  [unwired: 1 out]
            n677 = property on="魔王" class="Bool (strict)"() -> ("Left"=w1288:i32)  [unwired: 2 in, 2 out]
          }
        }
        n678 = case shown="\"speed\"" w1075 {
          tunnel: w1076 -> [w1260]
          tunnel: [w1258] -> w1069
          tunnel: [w1257] -> w1068
          tunnel: [w1241] -> w1037
          tunnel: w1039 -> [w1240]
          tunnel: w1039 -> [w1239]
          tunnel: w1038 -> [w1238]
          tunnel: w1038 -> [w1237]
          frame "speed" {
            n679 = Tick Count (ms)() -> (millisecond timer value=w1269:u32)
            n680 = property on="魔王" class="Bool (strict)"() -> ("Top"=w1261:i32)  [unwired: 2 in, 2 out]
            n681 = property on="魔王" class="Bool (strict)"() -> ("Top"=w1255:i32)  [unwired: 2 in, 2 out]
            n682 = Less?(x=w1255, y=0) -> (x < y?=w1253:bool)
            n683 = Greater?(x=w1240, y=400.0) -> (0:w1235:bool)
            n684 = Greater?(x=w1238, y=400.0) -> (0:w1244:bool)
            n685 = Less?(x=w1239, y=0.0) -> (x < y?=w1247:bool)
            n686 = Less?(x=w1237, y=0.0) -> (x < y?=w1248:bool)
            n687 = Greater?(x=w1261, y=400) -> (0:w1252:bool)
            n688 = Subtract(x=w1269, y=w1260) -> (x-y=w1268:u32)
            n689 = Or(x=w1252, y=w1253) -> (x .or. y?=w1251:bool)
            n690 = To Double Precision Float(number=w1268) -> (double precision float=w1267:dbl)
            n691 = And(x=w1235, y=w1244) -> (x .and. y?=w1249:bool)
            n692 = And(x=w1247, y=w1248) -> (x .and. y?=w1250:bool)
            n693 = Or(x=w1249, y=w1250) -> (x .or. y?=w1236:bool)
            n694 = local read "Å]Vy"() -> (w1256:i64)
            n695 = Divide(x=w1267, y=1000.0) -> (x/y=w1265:dbl)
            n696 = local read "Å]YÄ²"() -> (w1263:i32)
            n697 = case shown="True" w1236 {
              frame False {
              }
              frame True {
                w1270 = 200 ("x觸及位置")
                n698 = local write "Å]YÄ²"(w1270) -> ()
                n699 = Wait (ms)(milliseconds to wait=u32 100) -> ()  [unwired: 1 out]
                n700 = property on="魔王" class="Bool (strict)"("Top"=w1270) -> ()  [unwired: 2 in, 2 out]
              }
            }
            n701 = Multiply(x=w1265, y=w1256) -> (x*y=w1264:dbl)
            n702 = Add(x=w1264, y=w1263) -> (x+y=w1259:dbl)
            n703 = case shown="True" w1251 {
              tunnel: [enum16{"speed"}."speed" ("Enum") enum16{"speed"}."speed" ("Enum")] -> w1257
              tunnel: [w1272 w1279] -> w1258
              tunnel: w1260 -> [w1272 _]
              tunnel: w1259 -> [_ w1275]
              tunnel: w1256 -> [_ w1277]
              frame False {
              }
              frame True {
                n704 = Multiply(x=w1277, y=-1.0) -> (x*y=w1274:dbl)
                n705 = local write "Å]YÄ²"(w1275) -> ()
                n706 = Wait (ms)(milliseconds to wait=u32 25) -> ()  [unwired: 1 out]
                n707 = local write "Å]Vy"(w1274) -> ()
                n708 = Tick Count (ms)() -> (millisecond timer value=w1279:u32)
              }
            }
            n709 = property on="魔王" class="Bool (strict)"("Top"=w1259) -> ()  [unwired: 2 in, 2 out]
            n710 = Wait (ms)(milliseconds to wait=u32 10) -> ()  [unwired: 1 out]
            n711 = property on="魔王" class="Bool (strict)"() -> ("Top"=w1241:i32)  [unwired: 2 in, 2 out]
          }
        }
        n712 = case shown="\"speed\"" w1031 {
          tunnel: w1032 -> [w1213]
          tunnel: [w1211] -> w1030
          tunnel: [w1210] -> w1029
          tunnel: [w1194] -> w1028
          tunnel: w1027 -> [w1193]
          tunnel: w1027 -> [w1192]
          tunnel: w1026 -> [w1191]
          tunnel: w1026 -> [w1190]
          frame "speed" {
            n713 = Tick Count (ms)() -> (millisecond timer value=w1222:u32)
            n714 = property on="Y障礙 2" class="Bool (strict)"() -> ("Top"=w1214:i32)  [unwired: 2 in, 2 out]
            n715 = property on="Y障礙 2" class="Bool (strict)"() -> ("Top"=w1208:i32)  [unwired: 2 in, 2 out]
            n716 = Less?(x=w1208, y=0) -> (x < y?=w1206:bool)
            n717 = Greater?(x=w1193, y=400.0) -> (0:w1188:bool)
            n718 = Greater?(x=w1191, y=400.0) -> (0:w1197:bool)
            n719 = Less?(x=w1192, y=0.0) -> (x < y?=w1200:bool)
            n720 = Less?(x=w1190, y=0.0) -> (x < y?=w1201:bool)
            n721 = Greater?(x=w1214, y=400) -> (0:w1205:bool)
            n722 = Subtract(x=w1222, y=w1213) -> (x-y=w1221:u32)
            n723 = Or(x=w1205, y=w1206) -> (x .or. y?=w1204:bool)
            n724 = To Double Precision Float(number=w1221) -> (double precision float=w1220:dbl)
            n725 = And(x=w1188, y=w1197) -> (x .and. y?=w1202:bool)
            n726 = And(x=w1200, y=w1201) -> (x .and. y?=w1203:bool)
            n727 = Or(x=w1202, y=w1203) -> (x .or. y?=w1189:bool)
            n728 = local read "Vy 2"() -> (w1209:i32)
            n729 = local read "y觸及位置 2"() -> (w1216:i32)
            n730 = Divide(x=w1220, y=1000.0) -> (x/y=w1218:dbl)
            n731 = case shown="True" w1189 {
              frame False {
              }
              frame True {
                w1223 = 200 ("x觸及位置")
                n732 = local write "y觸及位置 2"(w1223) -> ()
                n733 = Wait (ms)(milliseconds to wait=u32 100) -> ()  [unwired: 1 out]
                n734 = property on="Y障礙 2" class="Bool (strict)"("Top"=w1223) -> ()  [unwired: 2 in, 2 out]
              }
            }
            n735 = Multiply(x=w1218, y=w1209) -> (x*y=w1217:dbl)
            n736 = Add(x=w1217, y=w1216) -> (x+y=w1212:dbl)
            n737 = case shown="True" w1204 {
              tunnel: [enum16{"speed"}."speed" ("Enum") enum16{"speed"}."speed" ("Enum")] -> w1210
              tunnel: [w1225 w1232] -> w1211
              tunnel: w1213 -> [w1225 _]
              tunnel: w1212 -> [_ w1228]
              tunnel: w1209 -> [_ w1230]
              frame False {
              }
              frame True {
                n738 = local write "y觸及位置 2"(w1228) -> ()
                n739 = Multiply(x=w1230, y=-1.0) -> (x*y=w1227:dbl)
                n740 = Wait (ms)(milliseconds to wait=u32 25) -> ()  [unwired: 1 out]
                n741 = local write "Vy 2"(w1227) -> ()
                n742 = Tick Count (ms)() -> (millisecond timer value=w1232:u32)
              }
            }
            n743 = property on="Y障礙 2" class="Bool (strict)"("Top"=w1212) -> ()  [unwired: 2 in, 2 out]
            n744 = Wait (ms)(milliseconds to wait=u32 10) -> ()  [unwired: 1 out]
            n745 = property on="Y障礙 2" class="Bool (strict)"() -> ("Top"=w1194:i32)  [unwired: 2 in, 2 out]
          }
        }
        n746 = case shown="\"speed\"" w1024 {
          tunnel: w1025 -> [w1166]
          tunnel: [w1164] -> w1023
          tunnel: [w1163] -> w1022
          tunnel: [w1147] -> w1021
          tunnel: w1020 -> [w1146]
          tunnel: w1020 -> [w1145]
          tunnel: w1019 -> [w1144]
          tunnel: w1019 -> [w1143]
          frame "speed" {
            n747 = Tick Count (ms)() -> (millisecond timer value=w1175:u32)
            n748 = property on="X障礙 2" class="Bool (strict)"() -> ("Left"=w1167:i32)  [unwired: 2 in, 2 out]
            n749 = property on="X障礙 2" class="Bool (strict)"() -> ("Left"=w1161:i32)  [unwired: 2 in, 2 out]
            n750 = Less?(x=w1161, y=0) -> (x < y?=w1159:bool)
            n751 = Greater?(x=w1146, y=500.0) -> (0:w1141:bool)
            n752 = Greater?(x=w1144, y=500.0) -> (0:w1150:bool)
            n753 = Less?(x=w1145, y=0.0) -> (x < y?=w1153:bool)
            n754 = Less?(x=w1143, y=0.0) -> (x < y?=w1154:bool)
            n755 = Greater?(x=w1167, y=500) -> (0:w1158:bool)
            n756 = Subtract(x=w1175, y=w1166) -> (x-y=w1174:u32)
            n757 = Or(x=w1158, y=w1159) -> (x .or. y?=w1157:bool)
            n758 = To Double Precision Float(number=w1174) -> (double precision float=w1173:dbl)
            n759 = And(x=w1141, y=w1150) -> (x .and. y?=w1155:bool)
            n760 = And(x=w1153, y=w1154) -> (x .and. y?=w1156:bool)
            n761 = Or(x=w1155, y=w1156) -> (x .or. y?=w1142:bool)
            n762 = local read "Vx 2"() -> (w1162:i32)
            n763 = local read "x觸及位置 2"() -> (w1169:i32)
            n764 = Divide(x=w1173, y=1000.0) -> (x/y=w1171:dbl)
            n765 = case shown="True" w1142 {
              frame False {
              }
              frame True {
                w1176 = 200 ("x觸及位置")
                n766 = local write "x觸及位置 2"(w1176) -> ()
                n767 = Wait (ms)(milliseconds to wait=u32 100) -> ()  [unwired: 1 out]
                n768 = property on="X障礙 2" class="Bool (strict)"("Left"=w1176) -> ()  [unwired: 2 in, 2 out]
              }
            }
            n769 = Multiply(x=w1171, y=w1162) -> (x*y=w1170:dbl)
            n770 = Add(x=w1170, y=w1169) -> (x+y=w1165:dbl)
            n771 = case shown="True" w1157 {
              tunnel: [enum16{"speed"}."speed" ("Enum") enum16{"speed"}."speed" ("Enum")] -> w1163
              tunnel: [w1178 w1185] -> w1164
              tunnel: w1166 -> [w1178 _]
              tunnel: w1165 -> [_ w1181]
              tunnel: w1162 -> [_ w1183]
              frame False {
              }
              frame True {
                n772 = local write "x觸及位置 2"(w1181) -> ()
                n773 = Multiply(x=w1183, y=-1.0) -> (x*y=w1180:dbl)
                n774 = Wait (ms)(milliseconds to wait=u32 25) -> ()  [unwired: 1 out]
                n775 = local write "Vx 2"(w1180) -> ()
                n776 = Tick Count (ms)() -> (millisecond timer value=w1185:u32)
              }
            }
            n777 = property on="X障礙 2" class="Bool (strict)"("Left"=w1165) -> ()  [unwired: 2 in, 2 out]
            n778 = Wait (ms)(milliseconds to wait=u32 10) -> ()  [unwired: 1 out]
            n779 = property on="X障礙 2" class="Bool (strict)"() -> ("Left"=w1147:i32)  [unwired: 2 in, 2 out]
          }
        }
        n780 = case shown="\"speed\"" w1138 {
          tunnel: w1139 -> [w1417]
          tunnel: [w1415] -> w1137
          tunnel: [w1414] -> w1136
          tunnel: [w1398] -> w1127
          tunnel: w1126 -> [w1397]
          tunnel: w1126 -> [w1396]
          tunnel: w1125 -> [w1395]
          tunnel: w1125 -> [w1394]
          frame "speed" {
            n781 = Tick Count (ms)() -> (millisecond timer value=w1426:u32)
            n782 = Greater?(x=w1397, y=400.0) -> (0:w1392:bool)
            n783 = Greater?(x=w1395, y=400.0) -> (0:w1401:bool)
            n784 = Less?(x=w1396, y=0.0) -> (x < y?=w1404:bool)
            n785 = Less?(x=w1394, y=0.0) -> (x < y?=w1405:bool)
            n786 = property on="Y障礙" class="Bool (strict)"() -> ("Top"=w1418:i32)  [unwired: 2 in, 2 out]
            n787 = property on="Y障礙" class="Bool (strict)"() -> ("Top"=w1412:i32)  [unwired: 2 in, 2 out]
            n788 = Less?(x=w1412, y=0) -> (x < y?=w1410:bool)
            n789 = Greater?(x=w1418, y=400) -> (0:w1409:bool)
            n790 = Subtract(x=w1426, y=w1417) -> (x-y=w1425:u32)
            n791 = Or(x=w1409, y=w1410) -> (x .or. y?=w1408:bool)
            n792 = And(x=w1392, y=w1401) -> (x .and. y?=w1406:bool)
            n793 = And(x=w1404, y=w1405) -> (x .and. y?=w1407:bool)
            n794 = To Double Precision Float(number=w1425) -> (double precision float=w1424:dbl)
            n795 = Or(x=w1406, y=w1407) -> (x .or. y?=w1393:bool)
            n796 = local read "Vy"() -> (w1413:i32)
            n797 = local read "y觸及位置"() -> (w1420:i32)
            n798 = Divide(x=w1424, y=1000.0) -> (x/y=w1422:dbl)
            n799 = case shown="True" w1393 {
              frame False {
              }
              frame True {
                w1427 = 200 ("y觸及位置")
                n800 = local write "y觸及位置"(w1427) -> ()
                n801 = Wait (ms)(milliseconds to wait=u32 100) -> ()  [unwired: 1 out]
                n802 = property on="Y障礙" class="Bool (strict)"("Top"=w1427) -> ()  [unwired: 2 in, 2 out]
              }
            }
            n803 = Multiply(x=w1422, y=w1413) -> (x*y=w1421:dbl)
            n804 = Add(x=w1421, y=w1420) -> (x+y=w1416:dbl)
            n805 = case shown="True" w1408 {
              tunnel: [enum16{"speed"}."speed" ("Enum") enum16{"speed"}."speed" ("Enum")] -> w1414
              tunnel: [w1429 w1436] -> w1415
              tunnel: w1417 -> [w1429 _]
              tunnel: w1416 -> [_ w1432]
              tunnel: w1413 -> [_ w1434]
              frame False {
              }
              frame True {
                n806 = local write "y觸及位置"(w1432) -> ()
                n807 = Multiply(x=w1434, y=-1.0) -> (x*y=w1431:dbl)
                n808 = Wait (ms)(milliseconds to wait=u32 25) -> ()  [unwired: 1 out]
                n809 = Tick Count (ms)() -> (millisecond timer value=w1436:u32)
                n810 = local write "Vy"(w1431) -> ()
              }
            }
            n811 = property on="Y障礙" class="Bool (strict)"("Top"=w1416) -> ()  [unwired: 2 in, 2 out]
            n812 = property on="Y障礙" class="Bool (strict)"() -> ("Top"=w1398:i32)  [unwired: 2 in, 2 out]
            n813 = Wait (ms)(milliseconds to wait=u32 10) -> ()  [unwired: 1 out]
          }
        }
        n814 = call-poly <vilib>:"Acquire Input Data.vi"("device ID"=w1135, "error in (no error)"=w1134) -> ("device ID"=w1107:refnum<k1>, "keys pressed"=w1133:T1, "error out"=w1106:errorcluster)  [unwired: 15 in]
        n815 = Increment(x=w1087) -> (x+1=w1088:i32)
        n816 = local write "遊玩時間"(w1088) -> ()
        n817 = Array To Cluster(array=w1133) -> (cluster=w1124:T2)
        n818 = Unbundle(w1124) -> ("keys pressed[0]"=w1132:T3)  [unwired: 8 out]
        n819 = case shown="\"A\"" w1132 {
          frame Default {
          }
          frame "A" {
            n820 = local read "X"() -> (w1389:dbl)
            n821 = Wait (ms)(milliseconds to wait=u32 10) -> ()  [unwired: 1 out]
            n822 = Add(x=-2.0, y=w1389) -> (x+y=w1387:dbl)
            n823 = local write "X"(w1387) -> ()
            n824 = property on="小精靈" class="Bool (strict)"("Left"=w1387) -> ()  [unwired: 2 in, 2 out]
          }
        }
        n825 = case shown="\"D\"" w1132 {
          frame Default {
          }
          frame "D" {
            n826 = local read "X"() -> (w1385:dbl)
            n827 = Wait (ms)(milliseconds to wait=u32 10) -> ()  [unwired: 1 out]
            n828 = Add(x=2.0, y=w1385) -> (x+y=w1383:dbl)
            n829 = local write "X"(w1383) -> ()
            n830 = property on="小精靈" class="Bool (strict)"("Left"=w1383) -> ()  [unwired: 2 in, 2 out]
          }
        }
        n831 = property on="Y障礙" class="Bool (strict)"() -> ("Top"=w1108:i32)  [unwired: 2 in, 2 out]
        n832 = property on="Y障礙" class="Bool (strict)"() -> ("Top"=w1114:i32)  [unwired: 2 in, 2 out]
        n833 = property on="Y障礙" class="Bool (strict)"() -> ("Left"=w1121:i32)  [unwired: 2 in, 2 out]
        n834 = property on="Y障礙" class="Bool (strict)"() -> ("Left"=w1119:i32)  [unwired: 2 in, 2 out]
        n835 = case shown="\"W\"" w1132 {
          frame Default {
          }
          frame "W" {
            n836 = local read "Y"() -> (w1381:dbl)
            n837 = Wait (ms)(milliseconds to wait=u32 10) -> ()  [unwired: 1 out]
            n838 = Add(x=-2.0, y=w1381) -> (x+y=w1379:dbl)
            n839 = local write "Y"(w1379) -> ()
            n840 = property on="小精靈" class="Bool (strict)"("Top"=w1379) -> ()  [unwired: 2 in, 2 out]
          }
        }
        n841 = case shown="\"S\"" w1132 {
          frame Default {
          }
          frame "S" {
            n842 = local read "Y"() -> (w1377:dbl)
            n843 = Wait (ms)(milliseconds to wait=u32 10) -> ()  [unwired: 1 out]
            n844 = Add(x=2.0, y=w1377) -> (x+y=w1375:dbl)
            n845 = local write "Y"(w1375) -> ()
            n846 = property on="小精靈" class="Bool (strict)"("Top"=w1375) -> ()  [unwired: 2 in, 2 out]
          }
        }
        n847 = local read "Y"() -> (w1122:dbl)
        n848 = local read "X"() -> (w1123:dbl)
        n849 = Add(x=w1121, y=17) -> (x+y=w1116:i32)
        n850 = Subtract(x=w1119, y=17) -> (x-y=w1117:i32)
        n851 = Subtract(x=w1114, y=15) -> (x-y=w1113:i32)
        n852 = Add(x=w1108, y=20) -> (x+y=w1109:i32)
        n853 = In Range and Coerce(upper limit=w1116, x=w1123, lower limit=w1117) -> (In Range?=w1112:bool)  [unwired: 1 out]
        n854 = In Range and Coerce(upper limit=w1109, x=w1122, lower limit=w1113) -> (In Range?=w1111:bool)  [unwired: 1 out]
        n855 = And(x=w1112, y=w1111) -> (x .and. y?=w1046:bool)
        n856 = property on="X障礙" class="Bool (strict)"() -> ("Top"=w1105:i32)  [unwired: 2 in, 2 out]
        n857 = property on="X障礙" class="Bool (strict)"() -> ("Top"=w1099:i32)  [unwired: 2 in, 2 out]
        n858 = property on="X障礙" class="Bool (strict)"() -> ("Left"=w1092:i32)  [unwired: 2 in, 2 out]
        n859 = property on="X障礙" class="Bool (strict)"() -> ("Left"=w1094:i32)  [unwired: 2 in, 2 out]
        n860 = local read "Y"() -> (w1091:dbl)
        n861 = property on="魔王" class="Bool (strict)"() -> ("Top"=w1052:i32)  [unwired: 2 in, 2 out]
        n862 = property on="魔王" class="Bool (strict)"() -> ("Top"=w1058:i32)  [unwired: 2 in, 2 out]
        n863 = property on="魔王" class="Bool (strict)"() -> ("Left"=w1065:i32)  [unwired: 2 in, 2 out]
        n864 = property on="魔王" class="Bool (strict)"() -> ("Left"=w1063:i32)  [unwired: 2 in, 2 out]
        n865 = local read "X"() -> (w1090:dbl)
        n866 = local read "Y"() -> (w1066:dbl)
        n867 = local read "X"() -> (w1067:dbl)
        n868 = property on="X障礙 2" class="Bool (strict)"() -> ("Top"=w1018:i32)  [unwired: 2 in, 2 out]
        n869 = property on="X障礙 2" class="Bool (strict)"() -> ("Top"=w1012:i32)  [unwired: 2 in, 2 out]
        n870 = property on="X障礙 2" class="Bool (strict)"() -> ("Left"=w1005:i32)  [unwired: 2 in, 2 out]
        n871 = property on="X障礙 2" class="Bool (strict)"() -> ("Left"=w1007:i32)  [unwired: 2 in, 2 out]
        n872 = property on="Y障礙 2" class="Bool (strict)"() -> ("Top"=w987:i32)  [unwired: 2 in, 2 out]
        n873 = property on="Y障礙 2" class="Bool (strict)"() -> ("Top"=w993:i32)  [unwired: 2 in, 2 out]
        n874 = property on="Y障礙 2" class="Bool (strict)"() -> ("Left"=w1000:i32)  [unwired: 2 in, 2 out]
        n875 = property on="Y障礙 2" class="Bool (strict)"() -> ("Left"=w998:i32)  [unwired: 2 in, 2 out]
        n876 = local read "X"() -> (w1086:dbl)
        n877 = local read "Y"() -> (w1085:dbl)
        n878 = Add(x=w1092, y=17) -> (x+y=w1097:i32)
        n879 = Subtract(x=w1094, y=17) -> (x-y=w1096:i32)
        n880 = Subtract(x=w1099, y=15) -> (x-y=w1100:i32)
        n881 = Add(x=w1105, y=20) -> (x+y=w1104:i32)
        n882 = local read "Y"() -> (w1004:dbl)
        n883 = local read "Y"() -> (w1001:dbl)
        n884 = local read "X"() -> (w1003:dbl)
        n885 = local read "X"() -> (w1002:dbl)
        n886 = Add(x=w1065, y=17) -> (x+y=w1060:i32)
        n887 = Subtract(x=w1063, y=17) -> (x-y=w1061:i32)
        n888 = Subtract(x=w1058, y=15) -> (x-y=w1057:i32)
        n889 = Add(x=w1052, y=20) -> (x+y=w1053:i32)
        n890 = In Range and Coerce(upper limit=w1097, x=w1090, lower limit=w1096) -> (In Range?=w1101:bool)  [unwired: 1 out]
        n891 = In Range and Coerce(upper limit=w1104, x=w1091, lower limit=w1100) -> (In Range?=w1102:bool)  [unwired: 1 out]
        n892 = In Range and Coerce(upper limit=40.0, x=w1086, lower limit=-20.0) -> (In Range?=w1084:bool)  [unwired: 1 out]
        n893 = In Range and Coerce(upper limit=25.0, x=w1085, lower limit=-18.0) -> (In Range?=w1083:bool)  [unwired: 1 out]
        n894 = Add(x=w1005, y=17) -> (x+y=w1010:i32)
        n895 = Subtract(x=w1007, y=17) -> (x-y=w1009:i32)
        n896 = Subtract(x=w1012, y=15) -> (x-y=w1013:i32)
        n897 = Add(x=w1000, y=17) -> (x+y=w995:i32)
        n898 = Subtract(x=w998, y=17) -> (x-y=w996:i32)
        n899 = Subtract(x=w993, y=15) -> (x-y=w992:i32)
        n900 = Add(x=w1018, y=20) -> (x+y=w1017:i32)
        n901 = Add(x=w987, y=20) -> (x+y=w988:i32)
        n902 = In Range and Coerce(upper limit=w1060, x=w1067, lower limit=w1061) -> (In Range?=w1056:bool)  [unwired: 1 out]
        n903 = In Range and Coerce(upper limit=w1053, x=w1066, lower limit=w1057) -> (In Range?=w1055:bool)  [unwired: 1 out]
        n904 = And(x=w1101, y=w1102) -> (x .and. y?=w1045:bool)
        n905 = And(x=w1084, y=w1083) -> (x .and. y?=w1043:bool)
        n906 = In Range and Coerce(upper limit=w1010, x=w1003, lower limit=w1009) -> (In Range?=w1014:bool)  [unwired: 1 out]
        n907 = In Range and Coerce(upper limit=w1017, x=w1004, lower limit=w1013) -> (In Range?=w1015:bool)  [unwired: 1 out]
        n908 = In Range and Coerce(upper limit=w995, x=w1002, lower limit=w996) -> (In Range?=w991:bool)  [unwired: 1 out]
        n909 = In Range and Coerce(upper limit=w988, x=w1001, lower limit=w992) -> (In Range?=w990:bool)  [unwired: 1 out]
        n910 = And(x=w1056, y=w1055) -> (x .and. y?=w1044:bool)
        n911 = And(x=w1014, y=w1015) -> (x .and. y?=w986:bool)
        n912 = And(x=w991, y=w990) -> (x .and. y?=w985:bool)
        n913 = Compound Arithmetic op=OR(w985, w986, w1033, w1034, w1035, w1036, w1043, w1051, w1050, w1049, w1048, w1047, w1046, w1045, w1044) -> (w1089:bool)
      }
      n914 = call-poly <vilib>:"Close Input Device.vi"("error in (no error)"=w976, "device ID"=w977) -> ()  [unwired: 8 in, 1 out]
      n915 = case shown="True" w965 {
        frame False {
          n916 = One Button Dialog(message="乖乖回去復健吧", button name ("OK")="爱") -> ()  [unwired: 1 out]
        }
        frame True {
          n917 = One Button Dialog(message="好像有點東西", button name ("OK")="再來啊!") -> ()  [unwired: 1 out]
        }
      }
    }
  }
  "終點" <- TRUE ("Boolean 3")
